vi "Tetra_TX-PROD_Payload.vi"(8 "error in":errorcluster, 10 "Input Constants":string[](array[string])=["18.75;1", "5;1", "COM4", "1", "1", "25", "0;0", "0;0", "1;20", "0", "0", "0", "", "10", "Z:\\State Files\\TEST2.csa", "", "3000", "4", "-10", "0.1", "", "", "C:\\RageATE\\Automated Tests\\Tetra WAM\\DVT\\Cal Files\\OUTPUT_CAL_080321-1118.csv"], 11 "Parameters":string[](array[string])=["skip", "18.75", "1", "5", "-1", "0", "5", "32.900000"]) -> (0 "error out":errorcluster, 2 "Payload Results":string[](array[string])=["-1.000", "-1.000", "32900.031", "-94.423", "-86.423", "-1.000", "16.450", "-1.000", "-1.000", "-1.000", "-1.000", "-1.000", "3.000", "-1.000", "-1.000", "15.000", "8.000", "8.000", "8.000", "-1.000", "-1.000", "-1.000", "-1.000", "-1.000", "-1.000", "-1.000", "-1.000", "-1.000", "-1.000", "-1.000", "-1.000", "-1.000", "-1.000", "-1.000", "-1.000", "-1.000", "-1.000", "-1.000", "-1.000", "-1.000", "-1.000", "-1.000", "-1.000", "-1.000", "0.504", "130.000", "-8.000", "32900.000", "-1.000", "-1.000", "P0027", "", "-1"])   [LabVIEW 2018]
uses:
  C:/RageATE-Tetra/Instruments/Ess Temp Plate/LabView Driver/Public/Watbus.dll
  Instruments/Ess Temp Plate/LabView Driver/Public/Watbus.dll
  8a334051-eedf-4406-ba3b-4766be56bf9e.vi
  458b4a15-084f-46bd-ad65-8d84519d0715.vi
  e7e3a4d5-9ed6-4285-8f90-f7af1205463a.vi
  778a857b-ea1c-4c41-85f0-8bde546241f8.vi
  765396e5-d7fa-4d1d-a6be-20604e030d46.vi
  35825170-2933-49a7-a6a3-6a45a8b9c174.vi
  498168d9-979f-4171-bbb2-b986919cd012.vi
  fd570da2-80e1-4258-b5ac-03cfe2f2c2d7.vi
  51f53847-2d88-46b1-9baf-ea88b261c08d.vi
  Infrastructure/Test Parameter Globals_1.0.0.vi
  Initialize References/Sequence Globals.vi
  Initialize References/Station References Global.vi
  Infrastructure/Test Result File Name Global.vi
  Tetra_Globals.vi
  <vilib>/Utility/file.llb/Write Delimited Spreadsheet (DBL).vi
  <vilib>/Utility/file.llb/Read Delimited Spreadsheet (DBL).vi
  Instruments/Agilent N5232A PNA-L/Labview Driver/Keysight PNA Series/Keysight PNA Series.lvlib
  Instruments/PNA/lib functions/Agilent ENA Series.lvlib
panel:
  out "result path":string
  out "adar_id":i32
  out "ser_rd":string
  out "AntiGlitch?(t)":bool
  in  "GetS11FromFile?(t)":bool=TRUE
  out "AVG_HARM":i32=4
  out "hx_fsl_corr":dbl=-1.0
  out "h2_fsl_corr":dbl=-1.0
  out "bypass ESA Freq Set(t)":bool
  out "TX-PASS?(T)":bool
  in  "Load_Prod_Limits(T)":bool=TRUE
  out "tx_flat_lim":dbl
  out "Tx_Flat":dbl
  out "resulting string":string
  out "TxFiltRead":bool
  out "x > 0?":bool
  in  "ess_error":errorcluster
  out "Freq Display":dbl=32.9 caption="Freq :  20"
  in  "Tab Control":T1(tab)
  out "MEAS_DCMON":bool
  out "CHIP_TEMP(t)":bool
  out "COMPORT":string="COM4"
  out "MODE":bool=TRUE
  out "Dist":dbl
  out "FILT_FCUT":dbl=25.0
  out "PLATE_TEMP(t)":bool
  out "MEAS_PS":bool
  out "MEAS_H2":bool=TRUE
  out "MEAS_Hx":bool=TRUE
  out "Hx_FREQ":dbl
  out "Hx_MULT":dbl
  out "H2_FREQ":dbl=40.0
  out "GANTRY(t)":bool=TRUE
  out "GET_DETECT":bool
  out "cmd;":string
  out "SOAK(m)":dbl
  out "Apply_FSL(t)":bool=TRUE
  out "MEAS_S11":bool
  out "S11_PORT":dbl
  out "comport":refnum<visa-resource-name>="COM4"
  out "AVG":i32=4
  out "ILabVIEW":refnum<k24>
  out "TEMP":dbl=25.0
  out "TX_PORT":i32=1
  out "V_SUPPLY":dbl=18.75
  out "EXT_ATT":dbl=5.0
  out "ADAR ATT":dbl
  out "TX_FILTER":i32=3
  out "REF_POW":dbl=5.0
  out "RF_FREQ":dbl=32.9
  out "TEMP(t)":bool
  out "V_SUPPLY(t)":bool
  out "TX_PORT(t)":bool
  out "REF_PWR(t)":bool
  out "TX_FILT(t)":bool
  out "ADAR_ATT(t)":bool
  out "EXT_ATT(t)":bool
  out "RF_FREQ(t)":bool=TRUE
  out "f_ref":dbl=16.45
  out "hx(t)":bool
  out "h2(t)":bool
  out "use-adar(t)":bool
  out "use-psa(t)":bool
  out "ps_meas(i)(w)":dbl[](array[numeric])=[-1.0, -1.0]
  out "rdv":dbl[](array[numeric])=[-1.0, -1.0, -1.0, -1.0, -1.0, -1.0, -1.0, -1.0, -1.0, -1.0]
  out "rdiv(i)":dbl[](array[numeric])=[-1.0, -1.0, -1.0, -1.0, -1.0, -1.0]
  out "rdiv(v)":dbl[](array[numeric])=[-1.0, -1.0, -1.0, -1.0, -1.0, -1.0]
  out "exa_mkr":dbl[](array[numeric])=[32900.0309, -94.423]
  out "h2_mkr":dbl[](array[numeric])=[-1.0, -1.0]
  out "Ampl_corr":dbl=-86.423
  out "s11":dbl=-1.0
  out "fsl_ampl_corr":dbl
  out "out_cal_ampl":dbl=-8.0
  out "out_cal freq":dbl=32900.0
  out "h2_dbc":dbl=-1.0
  out "hx_dbc":dbl
  out "hx_mkr":dbl[](array[numeric])
  out "fsl_corr_dB":dbl
  out "fsl(dB)":dbl
  out "hiband-flat":dbl
  out "lowband-flat":dbl
  out "h2_lim":dbl
  out "lowband-flat 2":dbl
  out "out_cal":dbl[][](array[numeric])=[[0.0, 0.0], [20000.0, -6.076], [20100.0, -6.075], [20200.0, -6.219], [20300.0, -6.234], [20400.0, -6.315], [20500.0, -6.131], [20600.0, -6.004], [20700.0, -6.283], [20800.0, -6.485], [20900.0, -6.42], [21000.0, -6.941], [21100.0, -6.789], [21200.0, -6.508], [21300.0, -6.41], [21400.0, -6.872], [21500.0, -6.938], [21600.0, -7.017], [21700.0, -7.269], [21800.0, -6.683], [21900.0, -6.297], [22000.0, -6.38], [22100.0, -6.432], [22200.0, -6.851], [22300.0, -6.503], [22400.0, -6.961], [22500.0, -6.827], [22600.0, -6.62], [22700.0, -6.74], [22800.0, -6.547], [22900.0, -6.559], [23000.0, -6.434], [23100.0, -6.642], [23200.0, -6.654], [23300.0, -6.563], [23400.0, -6.6], [23500.0, -6.836], [23600.0, -6.685], [23700.0, -6.139], [23800.0, -6.472], [23900.0, -6.849], [24000.0, -6.765], [24100.0, -6.802], [24200.0, -6.636], [24300.0, -6.397], [24400.0, -6.33], [24500.0, -6.799], [24600.0, -6.985], [24700.0, -7.181], [24800.0, -7.304], [24900.0, -7.242], [25000.0, -7.104], [25100.0, -7.249], [25200.0, -7.246], [25300.0, -7.161], [25400.0, -7.073], [25500.0, -7.471], [25600.0, -7.347], [25700.0, -7.254], [25800.0, -7.048], [25900.0, -7.016], [26000.0, -7.055], [26100.0, -7.436], [26200.0, -7.416], [26300.0, -7.406], [26400.0, -7.616], [26500.0, -7.56], [26600.0, -7.304], [26700.0, -7.165], [26800.0, -7.047], [26900.0, -7.196], [27000.0, -8.144], [27100.0, -7.775], [27200.0, -7.683], [27300.0, -8.261], [27400.0, -7.702], [27500.0, -7.067], [27600.0, -7.418], [27700.0, -7.363], [27800.0, -7.557], [27900.0, -8.241], [28000.0, -7.789], [28100.0, -7.932], [28200.0, -7.422], [28300.0, -7.539], [28400.0, -7.363], [28500.0, -7.293], [28600.0, -7.623], [28700.0, -7.8], [28800.0, -7.603], [28900.0, -7.302], [29000.0, -7.428], [29100.0, -7.212], [29200.0, -7.395], [29300.0, -7.337], [29400.0, -7.17], [29500.0, -7.328], [29600.0, -7.393], [29700.0, -7.363], [29800.0, -7.396], [29900.0, -7.295], [30000.0, -7.448], [30100.0, -7.434], [30200.0, -7.524], [30300.0, -7.411], [30400.0, -7.422], [30500.0, -7.643], [30600.0, -7.707], [30700.0, -7.612], [30800.0, -7.742], [30900.0, -7.916], [31000.0, -7.904], [31100.0, -8.064], [31200.0, -8.185], [31300.0, -8.079], [31400.0, -8.102], [31500.0, -8.357], [31600.0, -7.974], [31700.0, -8.361], [31800.0, -8.902], [31900.0, -8.745], [32000.0, -8.522], [32100.0, -8.392], [32200.0, -8.221], [32300.0, -7.885], [32400.0, -8.215], [32500.0, -8.486], [32600.0, -8.735], [32700.0, -8.287], [32800.0, -8.037], [32900.0, -8.0], [33000.0, -7.651], [33100.0, -7.755], [33200.0, -8.158], [33300.0, -8.086], [33400.0, -8.531], [33500.0, -8.093], [33600.0, -7.791], [33700.0, -7.841], [33800.0, -8.085], [33900.0, -7.787], [34000.0, -7.696], [34100.0, -8.068], [34200.0, -8.028], [34300.0, -7.958], [34400.0, -7.778], [34500.0, -8.182], [34600.0, -7.565], [34700.0, -7.759], [34800.0, -7.899], [34900.0, -7.536], [35000.0, -7.873], [35100.0, -8.126], [35200.0, -8.061], [35300.0, -7.731], [35400.0, -7.575], [35500.0, -7.802], [35600.0, -7.335], [35700.0, -7.39], [35800.0, -7.975], [35900.0, -7.981], [36000.0, -7.422], [36100.0, -7.632], [36200.0, -8.267], [36300.0, -7.907], [36400.0, -7.609], [36500.0, -7.858], [36600.0, -8.426], [36700.0, -8.44], [36800.0, -8.438], [36900.0, -8.536], [37000.0, -8.361], [37100.0, -8.731], [37200.0, -8.549], [37300.0, -8.609], [37400.0, -8.746], [37500.0, -9.42], [37600.0, -9.062], [37700.0, -8.792], [37800.0, -8.948], [37900.0, -8.893], [38000.0, -9.551], [38100.0, -9.086], [38200.0, -8.754], [38300.0, -8.61], [38400.0, -8.629], [38500.0, -8.895], [38600.0, -8.79], [38700.0, -8.437], [38800.0, -8.982], [38900.0, -8.564], [39000.0, -8.456], [39100.0, -8.944], [39200.0, -9.606], [39300.0, -9.246], [39400.0, -9.208], [39500.0, -9.78], [39600.0, -9.779], [39700.0, -9.292], [39800.0, -9.924], [39900.0, -9.871], [40000.0, -9.839]]
  out "h2_cal_ampl":dbl=-1.0
  out "h2_cal freq":dbl=-1.0
  out "h2_corr":dbl=-1.0
  out "h2_fsl_ampl_corr":dbl
  out "hx_cal_ampl":dbl=-1.0
  out "hx_cal freq":dbl=-1.0
  out "hx_fsl_ampl_corr":dbl
  out "hx_corr":dbl
  out "horn_Cal Freq Out":dbl
  out "horn_Ampl Out":dbl
  out "horn_cal":dbl[][](array[numeric])
  out "bpf":i32=1
  out "temp 0x":string="-1"
  out "detect":dbl=-1.0
  out "filt(num)":i32=3
  out "txatten-sel":i32=-1
  out "ext-atten(val)":dbl=-1.0
  out "adar-att(val)":dbl=-1.0
  out "iteration time(s)":dbl=91659.4314544 format="%_19f"
  out "relative seconds":dbl=91658.92763549999 format="%_19f"
  out "x-y":dbl=0.1592017999937525
  out "atten(code)ary (ro)":i32[](array[numeric])=[15, 8, 8, 8]
  out "plate_temp":sgl[](array[numeric])=[-1.0, -1.0] format="%.3g"
  out "temp_data":dbl[](array[numeric])
  out "readback":string
  out "dcw_lsl":dbl
  out "dcw_hsl":dbl
  out "pout_lsl":dbl
  out "pout_hsl":dbl
  out "s11_lsl":dbl
  out "s11_hsl":dbl
  out "FH_NOT(T)":bool
  out "no_fault":bool
  out "STOP(T)":bool
  out "pna-att":dbl=20.0
  out "do cmd?(f)":bool
  out "txp_#ofretries":i32
  # "Constants Locals Used in Payload"
  # "Index\tKey\tInput Constants\tUnits\n0\t1\tPS1-1 V;I\tVolt : Amp\n1\t1\tPS1-2 V:I\tVolt : Amp\n2\t1\tCOM PORT\tSTR\n3\t1\tMODE\tBool\n4\t1\tTXPORT;Antenna Dist\tant/inch\n5\t1\tTX Filt Cutoff\tGHz\n6\t1\tMeas Plate Temp; Meas Chip Temp\tBool;Bool\n7\t1\tMeas DC PS;Meas DCMON (Chip)\tBool;Bool\n8\t1\tMeas H2 \tBool;Freq(GHz)\n9\t1\tMeas H*x\tFreq(GHz);multiplier\n10\t1\tMeas S11;TXPORT\tBool;num\n11\t1\tRead Detector (1-4) \tBool\n12\t1\tcmd;…\tcmd;cmd\n13\t1\tTemp Soak Time\tmin\n14\t1\tPNA State File (local)\tPath\n15\t1\tENA State File\tPath\n16\t1\tENA RBW\tHz\n17\t1\tENA #of AVGs\tnum\n18\t1\tENA Ref Lvl\tdB\n19\t1\tENA Span\tMHz\n20\t1\tRFIN_CAL\tpath\n21\t1\tHORN_CAL\tpath\n22\t1\tOUTPUT_CAL\tpath\n23\t1\tFSL_APPLY\tbool\n24\t1\tDCW_LIMITS\tlsl;hsl\n25\t1\tPOUT_LIMITS\tlsl;hsl\n26\t1\tS11_LIMITS\tlsl;hsl"
  # "Input Parameters Locals"
  # "Update(t)"
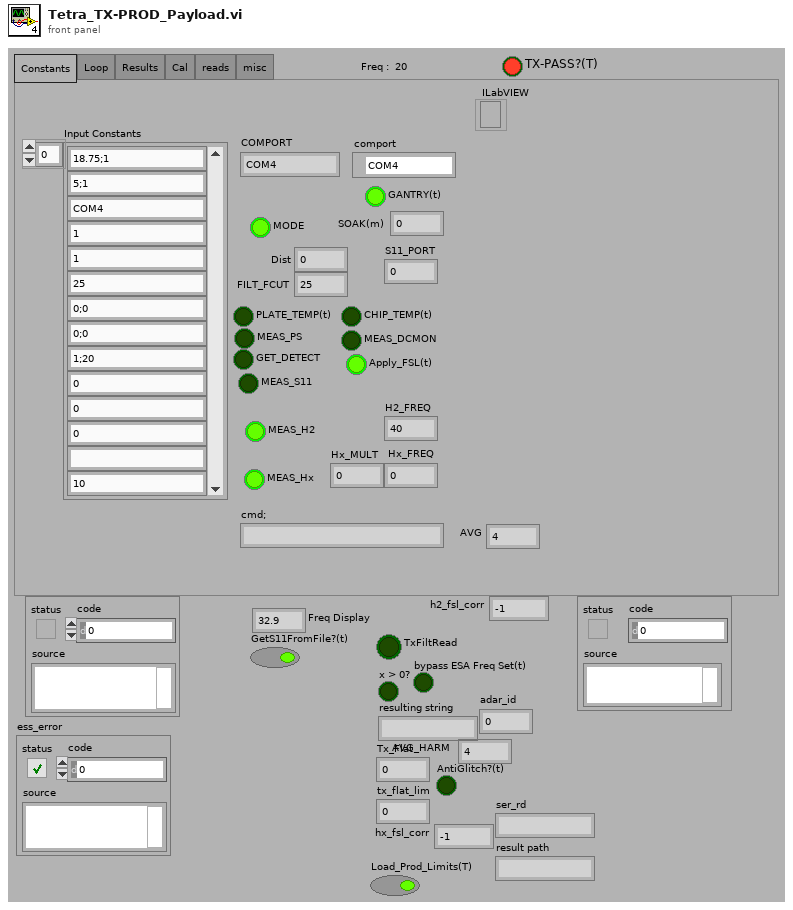
[diagram p1: front panel]
types:
  T1 = enum32{"Constants", "Loop", "Results", "Cal", "reads", "misc"}
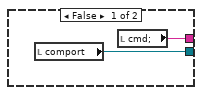
[diagram p3: hidden frame]
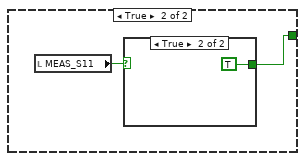
[diagram p4: hidden frame]
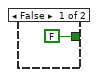
[diagram p5: hidden frame]
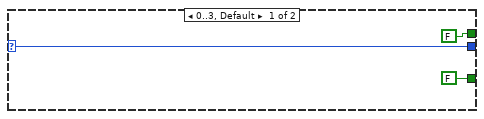
[diagram p6: hidden frame]
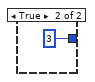
[diagram p7: hidden frame]
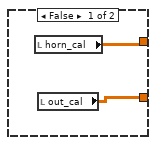
[diagram p8: hidden frame]
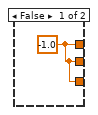
[diagram p9: hidden frame]
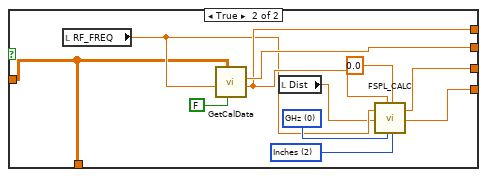
[diagram p10: hidden frame]
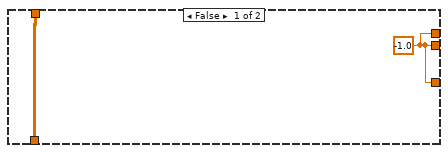
[diagram p11: hidden frame]
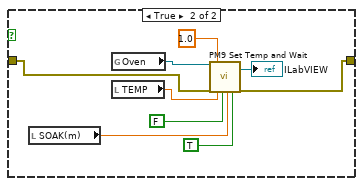
[diagram p12: hidden frame]
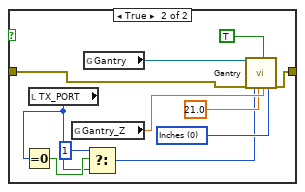
[diagram p13: hidden frame]
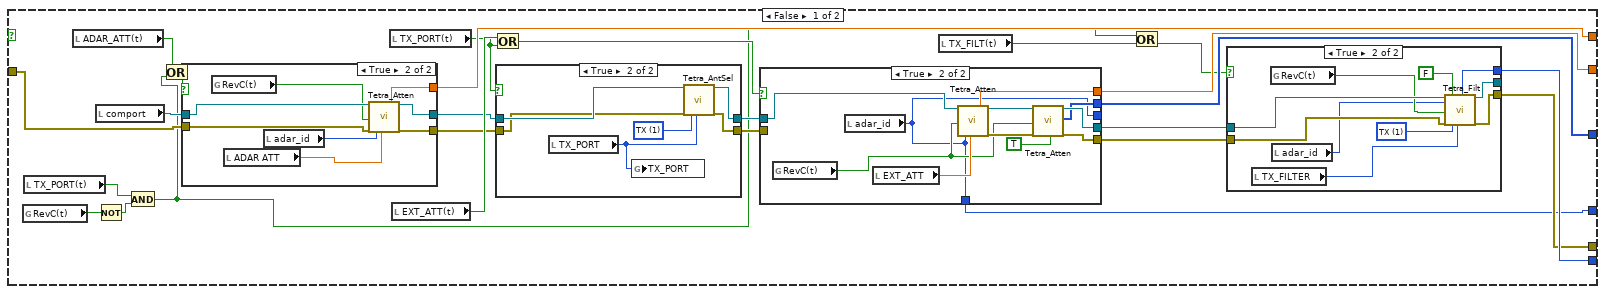
[diagram p15: hidden frame]
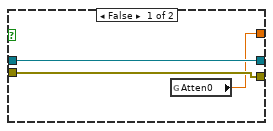
[diagram p17: hidden frame]
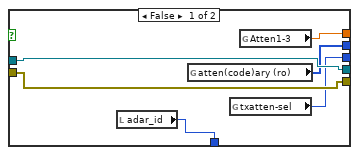
[diagram p18: hidden frame]
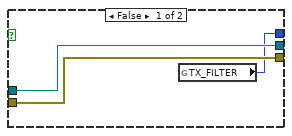
[diagram p19: hidden frame]
diagram:
  # "70\t1\tdc_hsl\tWatt\n71\t1\tdc_lsl\tWatt\n72\t1\tp_out_hsl\tdBm\n73\t1\tp_out_lsl\tdBm\n74\t1\ts11_hsl\tdb\n75\t1\ts11_lsl\tdb\n76\t1\th2_lim\tdbc\n77\t1\tdc|pout|s11|h2 (p/f)\t4b  bool \n78\t1\tpass/fail\tBool\n79\t1\tess_fault\tBool"
  n1 = flat-sequence {
    tunnel: ["error in"] -> w18
    tunnel: [w47] -> w20
    tunnel: [w46] -> w19
    tunnel: w18 -> [w44]
    tunnel: w20 -> [w1152]
    tunnel: w19 -> [w1132]
    tunnel: [w1152] -> w17
    tunnel: [w1132] -> w16
    tunnel: [w1145] -> w15
    tunnel: [w1144] -> w14
    tunnel: [w1143] -> w13
    tunnel: [w1151] -> w12
    tunnel: [w1150] -> w11
    tunnel: [w1149] -> w10
    tunnel: [w1148] -> w9
    tunnel: [w1147] -> w8
    tunnel: [w1146] -> w7
    tunnel: [w1142] -> w6
    tunnel: [w1141] -> w5
    tunnel: [w1130] -> w4
    tunnel: [w1129] -> w3
    tunnel: [w1128] -> w2
    tunnel: [w1127] -> w1
    tunnel: w17 -> [w1408]
    tunnel: w16 -> [w1395]
    tunnel: w15 -> [w1391]
    tunnel: w14 -> [w1406]
    tunnel: w13 -> [w1407]
    tunnel: w12 -> [w1405]
    tunnel: w11 -> [w1404]
    tunnel: w10 -> [w1403]
    tunnel: w9 -> [w1401]
    tunnel: w8 -> [w1400]
    tunnel: w7 -> [w1399]
    tunnel: w6 -> [w1402]
    tunnel: w5 -> [w1398]
    tunnel: w4 -> [w1393]
    tunnel: w3 -> [w1389]
    tunnel: w2 -> [w1386]
    tunnel: w1 -> [w1382]
    frame #0 {
      # "REV-C_TETRA_TX-PROD-DVT_LowRef"
      n2 = flat-sequence {
        frame #0 {
          w33 = TRUE ("Test Running (T)")
          n3 = global read "Station References Global.vi" "Gantry"() -> (w34:refnum<visa-resource-name>)
          n4 = call "WAM_ESS.vi"("VISA resource name"=w34, "error in (no error)"="ess_error", "Open Serial"=w33, "Test Running (T)"=w33, "Close Serial"=w33) -> ("FH_NOT(T)"=→"FH_NOT(T)":bool, "error out"=w31:errorcluster)  [unwired: 7 in, 2 out]
          n5 = local write "ess_error"(w31) -> ()
        }
      }
      n6 = global read "Test Result File Name Global.vi" "Test Results File Name"() -> (w22:path)
      n7 = First Call?() -> (First Call?: T/F=w23:bool)
      n8 = global read "Test Parameter Globals_1.0.0.vi" "Test Name"() -> (w28:string)
      n9 = And(x="Load_Prod_Limits(T)", y=w23) -> (x .and. y?=w25:bool)
      n10 = case shown="True" w25 {
        frame False {
        }
        frame True {
          n11 = global read "Sequence Globals.vi" "DevSupportPath"() -> (w38:path)
          n12 = global read "Sequence Globals.vi" "AppSupportPath 2"() -> (w40:path)
          n13 = global read "Sequence Globals.vi" "IsRuntime?"() -> (w41:bool)
          n14 = Build Path(base path=w38, name or relative path=path "3500007_TetraFinalTestAnalysis/testreport.ini" ("*.ini file")) -> (appended path=w36:path)
          n15 = Strip Path(path=w36) -> (name=w42:string)  [unwired: 1 out]
          n16 = Build Path(base path=w40, name or relative path=w42) -> (appended path=w39:path)
          n17 = Select(t=w39, s=w41, f=w36) -> (s? t:f=w43:path)
          n18 = call "ProdLimits.vi"("*.ini file"=w43) -> ()  [unwired: 9 in, 2 out]
        }
      }
      n19 = Path To String(path=w22) -> (string=→"result path":string)
      n20 = Equal?(x=w28, y="REV-C_TETRA_TX-PROD-DVT_LowRef") -> (x = y?=→"bypass ESA Freq Set(t)":bool)
      n21 = local write "TX-PASS?(T)"(FALSE ("TX-PASS?(T)")) -> ()
    }
    frame #1 {
      n22 = for {
        N: 2 -> [_]
        tunnel: [w58] -> w47
        tunnel: [w57] -> w46
        tunnel: w44 -> [w56]
        i -> [w53]
        stop <- w51 stop-if-true
        n23 = flat-sequence {
          tunnel: [w90] -> w89
          tunnel: ["Parameters"] -> w88
          tunnel: ["Input Constants"] -> w87
          tunnel: w56 -> [w90]
          tunnel: w89 -> [w95]
          tunnel: [w94] -> w86
          tunnel: w88 -> [w108]
          tunnel: w87 -> [w107]
          tunnel: [w106] -> w85
          tunnel: [w105] -> w84
          tunnel: [w104] -> w83
          tunnel: [w103] -> w82
          tunnel: [w102] -> w81
          tunnel: [w100] -> w80
          tunnel: [w101] -> w79
          tunnel: [w99] -> w78
          tunnel: [w98] -> w77
          tunnel: [w97] -> w76
          tunnel: w86 -> [w250]
          tunnel: [w250] -> w75
          tunnel: w85 -> [w249]
          tunnel: w84 -> [w246]
          tunnel: w83 -> [w234]
          tunnel: w82 -> [w229]
          tunnel: w81 -> [w243]
          tunnel: w80 -> [w242]
          tunnel: w79 -> [w240]
          tunnel: w78 -> [w237]
          tunnel: w77 -> [w235]
          tunnel: w76 -> [w227]
          tunnel: w75 -> [w303]
          tunnel: [w302] -> w74
          tunnel: [w383] -> w73
          tunnel: w74 -> [w382]
          tunnel: w73 -> [w399]
          tunnel: [w399] -> w72
          tunnel: w72 -> [w401]
          tunnel: [w401] -> w55
          tunnel: [w419] -> w71
          tunnel: w55 -> [w419]
          tunnel: w71 -> [w420]
          tunnel: [w421] -> w70
          tunnel: w70 -> [w433]
          tunnel: [w433] -> w69
          tunnel: [w432] -> w68
          tunnel: [w436] -> w67
          tunnel: w69 -> [w435]
          tunnel: w68 -> [w434]
          tunnel: [w434] -> w66
          tunnel: w67 -> [w604]
          tunnel: [w603] -> w65
          tunnel: w66 -> [w608]
          tunnel: [w617] -> w64
          tunnel: w65 -> [w616]
          tunnel: w64 -> [w641]
          tunnel: [w641] -> w63
          tunnel: w63 -> [w647]
          tunnel: [w642] -> w62
          tunnel: [w901] -> w61
          tunnel: w62 -> [w903]
          tunnel: w61 -> [w1004]
          tunnel: [w1004] -> w60
          tunnel: [w1006] -> w59
          tunnel: w60 -> [w1005]
          tunnel: w59 -> [w1037]
          tunnel: [w1037] -> w49
          tunnel: [w1036] -> w54
          tunnel: w49 -> [w1062]
          tunnel: [w1061] -> w48
          tunnel: [w1092] -> w58
          tunnel: w48 -> [w1079]
          tunnel: [w1080] -> w57
          tunnel: [w1081] -> w50
          frame #0 {
            n24 = call <vilib>:"High Resolution Relative Seconds.vi"() -> ("relative seconds"=→"relative seconds":dbl)
          }
          frame #1 {
            n25 = flat-sequence {
              tunnel: w107 -> [w212]
              tunnel: [w181] -> w97
              frame #0 {
                w140 = ";" ("regular expression")
                # "Get the Test Constants"
                n26 = Index Array(array=w212, index #1=2 ("index"), index #3=4 ("index"), index #8=10 ("index"), index #10=17 ("index"), index #11=20 ("index"), index #12=9 ("index"), index #13=13 ("index"), index #14=23 ("index")) -> (element #1=→"COMPORT":string, element #2=w187:string, element #3=w163:string, element #4=w202:string, element #5=w206:string, element #6=w205:string, element #7=w196:string, element #8=w185:string, element #9=w197:string, element #10=w141:string, element #12=w179:string, element #13=w168:string, element #14=w164:string, element #15=w155:string, element #16=w158:string, element #17=w150:string, element #18=w144:string, element #19=w143:string, element #20=→"ser_rd":string)  [unwired: 12 in, 1 out]
                n27 = call "StringToNumberControlWithBool.vi"("String In"=w187) -> ("NOT = 0"=→"MODE":bool)  [unwired: 7 in, 1 out]
                n28 = call "StringToNumberControlWithBool.vi"("String In"=w202) -> ("Number Out"=→"FILT_FCUT":dbl)  [unwired: 7 in, 1 out]
                n29 = call "StringToNumberControlWithBool.vi"("String In"=w197) -> ("NOT = 0"=→"GET_DETECT":bool)  [unwired: 7 in, 1 out]
                n30 = call "StringToNumberControlWithBool(x2).vi"("Seperator"=w140, "string"=w141) -> ("Num(2)"=→"AVG_HARM":dbl, "Num"=→"AVG":dbl)  [unwired: 3 in, 5 out]
                n31 = call "StringToNumberControlWithBool.vi"("String In"=w168) -> ("Number Out"=→"SOAK(m)":dbl)  [unwired: 7 in, 1 out]
                n32 = call "StringToNumberControlWithBool.vi"("String In"=w143) -> ("Number Out"=→"tx_flat_lim":dbl)  [unwired: 7 in, 1 out]
                n33 = call <vilib>:"Trim Whitespace.vi"("string"=w179) -> ("trimmed string"=w175:string)  [unwired: 1 in]
                n34 = Match Pattern(string=w163, regular expression=";") -> (before substring=w162:string, after substring=w160:string)  [unwired: 1 in, 2 out]
                n35 = Match Pattern(string=w206, regular expression=";") -> (before substring=w210:string, after substring=w209:string)  [unwired: 1 in, 2 out]
                n36 = Match Pattern(string=w205, regular expression=";") -> (before substring=w218:string, after substring=w217:string)  [unwired: 1 in, 2 out]
                n37 = Match Pattern(string=w196, regular expression=";") -> (before substring=w194:string, after substring=w192:string)  [unwired: 1 in, 2 out]
                n38 = Match Pattern(string=w185, regular expression=w140) -> (before substring=w184:string, after substring=w182:string)  [unwired: 1 in, 2 out]
                n39 = call "StringToNumberControlWithBool(x2).vi"("Seperator"=";" ("regular expression"), "string"=w155) -> ("Num(2)"=→"dcw_hsl":dbl, "Num"=→"dcw_lsl":dbl, "Seperator Out"=w151:string)  [unwired: 3 in, 4 out]
                n40 = Empty String/Path?(string/path=w182) -> (empty?=w181:bool)
                n41 = call "StringToNumberControlWithBool.vi"("String In"=w162) -> ("NOT = 0"=→"GANTRY(t)":bool)  [unwired: 7 in, 1 out]
                n42 = call "StringToNumberControlWithBool.vi"("String In"=w160) -> ("Number Out"=→"Dist":dbl)  [unwired: 7 in, 1 out]
                n43 = call "StringToNumberControlWithBool.vi"("String In"=w210) -> ("NOT = 0"=→"PLATE_TEMP(t)":bool)  [unwired: 7 in, 1 out]
                n44 = call "StringToNumberControlWithBool.vi"("String In"=w209) -> ("NOT = 0"=→"CHIP_TEMP(t)":bool)  [unwired: 7 in, 1 out]
                n45 = call "StringToNumberControlWithBool.vi"("String In"=w218) -> ("NOT = 0"=→"MEAS_PS":bool)  [unwired: 7 in, 1 out]
                n46 = call "StringToNumberControlWithBool.vi"("String In"=w217) -> ("NOT = 0"=→"MEAS_DCMON":bool)  [unwired: 7 in, 1 out]
                n47 = call "StringToNumberControlWithBool.vi"("String In"=w194) -> ("NOT = 0"=→"MEAS_H2":bool)  [unwired: 7 in, 1 out]
                n48 = call "StringToNumberControlWithBool.vi"("String In"=w192) -> ("Number Out"=→"H2_FREQ":dbl)  [unwired: 7 in, 1 out]
                n49 = call "StringToNumberControlWithBool.vi"("String In"=w184) -> ("NOT = 0"=→"MEAS_S11":bool)  [unwired: 7 in, 1 out]
                n50 = call "StringToNumberControlWithBool.vi"("String In"=w182) -> ("Number Out"=→"S11_PORT":dbl)  [unwired: 7 in, 1 out]
                n51 = call "StringToNumberControlWithBool(x2).vi"("Seperator"=w151, "string"=w158) -> ("Num(2)"=→"pout_hsl":dbl, "Num"=→"pout_lsl":dbl, "Seperator Out"=w149:string)  [unwired: 3 in, 4 out]
                n52 = Match Pattern(string=w175, regular expression=";") -> (before substring=w178:string, after substring=w177:string)  [unwired: 1 in, 2 out]
                n53 = call "StringToNumberControlWithBool.vi"("String In"=w178) -> ("Number Out"=→"Hx_FREQ":dbl, "NOT = 0"=w174:bool)  [unwired: 7 in]
                n54 = call "StringToNumberControlWithBool.vi"("String In"=w177) -> ("Number Out"=→"Hx_MULT":dbl, "NOT = 0"=w173:bool)  [unwired: 7 in]
                n55 = call "StringToNumberControlWithBool(x2).vi"("Seperator"=w149, "string"=w150) -> ("Num(2)"=→"s11_hsl":dbl, "Num"=→"s11_lsl":dbl, "Seperator Out"=w146:string)  [unwired: 3 in, 4 out]
                n56 = And(x=w174, y=w173) -> (x .and. y?=→"MEAS_Hx":bool)
                n57 = call "StringToNumberControlWithBool(x2).vi"("Seperator"=w146, "string"=w144) -> ("Num"=→"h2_lim":dbl)  [unwired: 3 in, 6 out]
                n58 = call "StringToNumberControlWithBool.vi"("String In"=w164) -> ("NOT = 0"=→"Apply_FSL(t)":bool)  [unwired: 7 in, 1 out]
              }
            }
            n59 = control-ref of="Freq Display"() -> (w96:refnum<vi>)
            n60 = flat-sequence {
              tunnel: w108 -> [w135]
              tunnel: [w113] -> w106
              tunnel: [w112] -> w105
              tunnel: [w134] -> w104
              tunnel: [w133] -> w103
              tunnel: [w132] -> w102
              tunnel: [w131] -> w101
              tunnel: [w130] -> w100
              tunnel: [w128] -> w99
              tunnel: [w109] -> w98
              tunnel: w96 -> [w123]
              tunnel: w95 -> [w120]
              tunnel: [w119] -> w94
              frame #0 {
                # "Get the Test Parameters"
                n61 = Index Array(array=w135) -> (element #1=w130:string, element #2=w137:string, element #3=w136:string, element #4=w127:string, element #5=w126:string, element #6=w125:string, element #7=w118:string, element #8=w110:string)  [unwired: 9 in, 1 out]
                n62 = call "TempControlWithBool.vi"("INPUT"=w130) -> ("out"=→"TEMP":dbl, "Valid(t)"=w128:bool)  [unwired: 6 in, 1 out]
                n63 = Fract/Exp String To Number(string=w137) -> (number=w132:dbl)  [unwired: 3 in, 1 out]
                "V_SUPPLY" <- w132
                n64 = Decimal String To Number(string=w136) -> (number=w133:i32)  [unwired: 2 in, 1 out]
                "TX_PORT" <- w133
                n65 = Fract/Exp String To Number(string=w127) -> (number=w131:dbl)  [unwired: 3 in, 1 out]
                "REF_POW" <- w131
                n66 = Decimal String To Number(string=w126) -> (number=w134:i32)  [unwired: 2 in, 1 out]
                "TX_FILTER" <- w134
                n67 = Fract/Exp String To Number(string=w125) -> (number=w112:dbl)  [unwired: 3 in, 1 out]
                "ADAR ATT" <- w112
                n68 = Fract/Exp String To Number(string=w118) -> (number=w113:dbl)  [unwired: 3 in, 1 out]
                "EXT_ATT" <- w113
                n69 = Fract/Exp String To Number(string=w110) -> (number=w109:dbl)  [unwired: 3 in, 1 out]
                "RF_FREQ" <- w109
                "Freq Display" <- w109
                n70 = Concatenate Strings("Freq :  " ("string"), w110) -> (w122:string)
                n71 = Divide(x=w109, y=2.0) -> (x/y=→"f_ref":dbl)
                n72 = Not Equal?(x=w112, y=-1.0) -> (x != y?=→"use-adar(t)":bool)
                n73 = Not Equal?(x=w113, y=-1.0) -> (x != y?=→"use-psa(t)":bool)
                n74 = property class="DigNum (strict)"(reference=w123, error in=w120, "Caption.Text"=w122) -> (error out=w119:errorcluster)  [unwired: 1 out]
              }
            }
          }
          frame #2 {
            # "Check if value changed\nif value changed (t) use to skip the routine"
            n75 = call "Is Value Changed.vim"("value"=w242) -> ("changed or first call?"=w239:bool)
            n76 = call "Is Value Changed.vim"("value"=w243) -> ("changed or first call?"=→"V_SUPPLY(t)":bool)
            n77 = call "Is Value Changed.vim"("value"=w229) -> ("changed or first call?"=→"TX_PORT(t)":bool)
            n78 = call "Is Value Changed.vim"("value"=w240) -> ("changed or first call?"=→"REF_PWR(t)":bool)
            n79 = call "Is Value Changed.vim"("value"=w246) -> ("changed or first call?"=→"ADAR_ATT(t)":bool)
            n80 = call "Is Value Changed.vim"("value"=w249) -> ("changed or first call?"=→"EXT_ATT(t)":bool)
            n81 = call "Is Value Changed.vim"("value"=w235) -> ("changed or first call?"=→"RF_FREQ(t)":bool)
            n82 = flat-sequence {
              frame #0 {
                # "Setup the H2 measurement"
                n83 = local read "RF_FREQ"() -> (w280:dbl)
                n84 = local read "H2_FREQ"() -> (w276:dbl)
                n85 = local read "MEAS_H2"() -> (w277:bool)
                n86 = Equal?(x=w276, y=w280) -> (x = y?=w279:bool)
                n87 = Multiply(x=w276, y=2.0) -> (x*y=w274:dbl)
                n88 = And(x=w279, y=w277) -> (x .and. y?=→"h2(t)":bool)
                n89 = local write "H2_FREQ"(w274) -> ()
              }
            }
            n90 = case shown="-1" w234 {
              selector: w234 -> [w283 _]
              tunnel: [w283 w286] -> w233
              tunnel: [FALSE ("changed or first call?") w285] -> w230
              tunnel: [FALSE ("TxFiltRead") TRUE ("TxFiltRead")] -> w222
              frame 0..3, Default {
              }
              frame -1 {
                n91 = local read "FILT_FCUT"() -> (w288:dbl)
                n92 = local read "RF_FREQ"() -> (w289:dbl)
                n93 = Greater Or Equal?(x=w289, y=w288) -> (x >= y?=w287:bool)
                n94 = case shown="False" w287 {
                  tunnel: [2 3] -> w286
                  frame False {
                  }
                  frame True {
                  }
                }
                n95 = call "Is Value Changed.vim"("value"=w286) -> ("changed or first call?"=w285:bool)
              }
            }
            "TxFiltRead" <- w222
            n96 = flat-sequence {
              frame #0 {
                # "Setup the H*X measurement"
                n97 = local read "RF_FREQ"() -> (w264:dbl)
                n98 = local read "Hx_MULT"() -> (w258:dbl)
                n99 = local read "Hx_FREQ"() -> (w260:dbl)
                n100 = local read "MEAS_Hx"() -> (w261:bool)
                n101 = Multiply(x=w260, y=w258) -> (x*y=w259:dbl)
                n102 = Equal?(x=w260, y=w264) -> (x = y?=w263:bool)
                n103 = And(x=w263, y=w261) -> (x .and. y?=→"hx(t)":bool)
                n104 = local write "Hx_FREQ"(w259) -> ()
              }
            }
            n105 = local read "MEAS_S11"() -> (w225:bool)
            n106 = First Call?() -> (First Call?: T/F=w223:bool)
            n107 = case shown="True" w223 {
              tunnel: [w252 w257] -> w220
              tunnel: [w251 w253] -> w224
              frame False {
                n108 = local read "comport"() -> (w251:refnum<visa-resource-name>)
                n109 = local read "cmd;"() -> (w252:string)
              }
              frame True {
                n110 = local read "COMPORT"() -> (w254:string)
                n111 = global read "Tetra_Globals.vi" "comport"() -> (w255:refnum<visa-resource-name>)
                n112 = Empty String/Path?(string/path=w254) -> (empty?=w256:bool)
                n113 = Select(t=w255, s=w256, f=w254) -> (s? t:f=w253:refnum<visa-resource-name>)
                n114 = global read "Tetra_Globals.vi" "cmd;"() -> (w257:string)
              }
            }
            "cmd;" <- w220
            "comport" <- w224
            n115 = And(x=w239, y=w237) -> (x .and. y?=→"TEMP(t)":bool)
            n116 = And(x=w227, y=w225) -> (x .and. y?=w226:bool)
            n117 = case shown="False" w226 {
              tunnel: w229 -> [w269 _]
              tunnel: [w265 w271] -> w228
              frame False {
                n118 = local read "S11_PORT"() -> (w268:dbl)
                n119 = local read "MEAS_S11"() -> (w266:bool)
                n120 = Equal?(x=w268, y=w269) -> (x = y?=w267:bool)
                n121 = And(x=w266, y=w267) -> (x .and. y?=w265:bool)
              }
              frame True {
                n122 = local read "MEAS_S11"() -> (w270:bool)
                n123 = case shown="True" w270 {
                  tunnel: [FALSE TRUE] -> w271
                  frame False {
                  }
                  frame True {
                  }
                }
              }
            }
            n124 = call "Is Value Changed.vim"("value"=w234) -> ("changed or first call?"=w231:bool)
            n125 = Empty String/Path?(string/path=w220) -> (empty?=→"do cmd?(f)":bool)
            n126 = Or(x=w230, y=w231) -> (x .or. y?=→"TX_FILT(t)":bool)
            n127 = local write "TX_FILTER"(w233) -> ()
            n128 = local write "MEAS_S11"(w228) -> ()
          }
          frame #3 {
            n129 = flat-sequence "CALIBRATION TABLES" {
              tunnel: [w325] -> w302
              tunnel: w303 -> [w326]
              tunnel: [w304] -> w301
              tunnel: [w320] -> w300
              tunnel: [w319] -> w299
              tunnel: [w318] -> w298
              tunnel: [w317] -> w297
              tunnel: [w316] -> w296
              tunnel: [w315] -> w295
              tunnel: [w314] -> w294
              tunnel: [w313] -> w293
              tunnel: [w312] -> w292
              frame #0 {
                n130 = First Call?() -> (First Call?: T/F=w305:bool)
                n131 = case shown="True" w305 {
                  tunnel: [w331 w334] -> w322
                  tunnel: [w332 w333] -> w311
                  frame False {
                    n132 = local read "horn_cal"() -> (w332:dbl[][])
                    n133 = local read "out_cal"() -> (w331:dbl[][])
                  }
                  frame True {
                    n134 = global read "Tetra_Globals.vi" "HORN_CAL"() -> (w333:dbl[][])
                    n135 = global read "Tetra_Globals.vi" "OUT_CAL"() -> (w334:dbl[][])
                  }
                }
                "out_cal" <- w322
                "horn_cal" <- w311
                n136 = local read "RF_FREQ"() -> (w330:dbl)
                n137 = Multiply(x=w330, y=1000.0) -> (x*y=w329:dbl)
                n138 = call "GetCalData.vi"("Open new file T"=FALSE, "Ary In"=w322, "error in (no error)"=w326, "RF Freq (MHz)"=w329) -> ("error out"=w325:errorcluster, "Ampl Out"=→"out_cal_ampl":dbl, "Cal Freq Out"=→"out_cal freq":dbl, "array out"=w321:dbl[][])  [unwired: 2 in, 2 out]
                n139 = local read "Apply_FSL(t)"() -> (w308:bool)
                n140 = local read "MEAS_Hx"() -> (w306:bool)
                n141 = local read "MEAS_H2"() -> (w307:bool)
                n142 = case shown="False" w308 {
                  tunnel: [-1.0 ("Cal Freq Out") w363] -> w312
                  tunnel: [w352 w362] -> w313
                  tunnel: w311 -> [w351 w354]
                  tunnel: [w352 w358] -> w314
                  tunnel: [w352 w356] -> w315
                  tunnel: [w351 w354] -> w309
                  frame False {
                    w352 = 0.0 ("Ampl Out")
                  }
                  frame True {
                    w359 = u16 2 items=["Meter", "Feet", "Inches"] ("d(units)")
                    w361 = u16 0 items=["GHz", "MHz"] ("f(units)")
                    n143 = local read "RF_FREQ"() -> (w357:dbl)
                    n144 = call "GetCalData.vi"("Open new file T"=FALSE, "Ary In"=w354, "RF Freq (MHz)"=w357) -> ("Ampl Out"=w362:dbl, "Cal Freq Out"=w363:dbl)  [unwired: 3 in, 4 out]
                    n145 = local read "Dist"() -> (w355:dbl)
                    n146 = call "FSPL_CALC.vi"("f"=w357, "d"=w355, "Ant1 Gain (dB)"=w362, "f(units)"=w361, "Ant2 Gain dB"=0.0 ("Ant1 Gain (dB)"), "d(units)"=w359) -> ("Corr(dB)"=w358:dbl, "fsl(dB)"=w356:dbl)  [unwired: 11 in, 1 out]
                  }
                }
                n147 = case shown="True" w307 {
                  tunnel: [w366 w381] -> w316
                  tunnel: [w366 w380] -> w317
                  tunnel: w321 -> [_ w378]
                  tunnel: [w366 w370] -> w320
                  tunnel: w309 -> [w365 w367]
                  tunnel: [w365 w367] -> w310
                  frame False {
                    w366 = -1.0 ("Ampl Out")
                  }
                  frame True {
                    w373 = u16 2 items=["Meter", "Feet", "Inches"] ("d(units)")
                    w374 = u16 0 items=["GHz", "MHz"] ("f(units)")
                    n148 = local read "H2_FREQ"() -> (w371:dbl)
                    n149 = call "GetCalData.vi"("Open new file T"=FALSE, "Ary In"=w367, "RF Freq (MHz)"=w371) -> ("Ampl Out"=w369:dbl)  [unwired: 3 in, 5 out]
                    n150 = local read "Dist"() -> (w375:dbl)
                    n151 = Multiply(x=1000.0 ("y"), y=w371) -> (x*y=w379:dbl)
                    n152 = call "GetCalData.vi"("Open new file T"=FALSE, "Ary In"=w378, "RF Freq (MHz)"=w379) -> ("Ampl Out"=w380:dbl, "Cal Freq Out"=w381:dbl)  [unwired: 3 in, 4 out]
                    n153 = call "FSPL_CALC.vi"("f"=w371, "d"=w375, "Ant1 Gain (dB)"=w369, "f(units)"=w374, "Ant2 Gain dB"=0.0, "d(units)"=w373) -> ("Corr(dB)"=w370:dbl)  [unwired: 11 in, 2 out]
                  }
                }
                n154 = case shown="True" w306 {
                  tunnel: [w335 w350] -> w318
                  tunnel: [w335 w349] -> w319
                  tunnel: w321 -> [_ w347]
                  tunnel: [w335 w339] -> w304
                  tunnel: w310 -> [_ w336]
                  frame False {
                    w335 = -1.0 ("Ampl Out")
                  }
                  frame True {
                    w342 = u16 2 items=["Meter", "Feet", "Inches"] ("d(units)")
                    w343 = u16 0 items=["GHz", "MHz"] ("f(units)")
                    n155 = local read "Hx_FREQ"() -> (w340:dbl)
                    n156 = call "GetCalData.vi"("Open new file T"=FALSE, "Ary In"=w336, "RF Freq (MHz)"=w340) -> ("Ampl Out"=w338:dbl)  [unwired: 3 in, 5 out]
                    n157 = local read "Dist"() -> (w344:dbl)
                    n158 = Multiply(x=1000.0 ("y"), y=w340) -> (x*y=w348:dbl)
                    n159 = call "GetCalData.vi"("Open new file T"=FALSE, "Ary In"=w347, "RF Freq (MHz)"=w348) -> ("Ampl Out"=w349:dbl, "Cal Freq Out"=w350:dbl)  [unwired: 3 in, 4 out]
                    n160 = call "FSPL_CALC.vi"("f"=w340, "d"=w344, "Ant1 Gain (dB)"=w338, "f(units)"=w343, "Ant2 Gain dB"=0.0, "d(units)"=w342) -> ("Corr(dB)"=w339:dbl)  [unwired: 11 in, 2 out]
                  }
                }
              }
            }
            "h2_cal freq" <- w296
            "h2_cal_ampl" <- w297
            "hx_cal freq" <- w298
            "hx_cal_ampl" <- w299
            "h2_fsl_corr" <- w300
            "hx_fsl_corr" <- w301
            "horn_Cal Freq Out" <- w292
            "horn_Ampl Out" <- w293
            "fsl_corr_dB" <- w294
            "fsl(dB)" <- w295
          }
          frame #4 {
            n161 = flat-sequence {
              tunnel: [w387] -> w383
              tunnel: w382 -> [w386]
              frame #0 {
                # "3-23-22\nneed to add bypass if ess is tripped so it wont set the temperature and soak"
                # "Set The Temperature"
                n162 = global read "Station References Global.vi" "Oven Present?"() -> (w384:bool)
                n163 = local read "TEMP(t)"() -> (w388:bool)
                n164 = And(x=w388, y=w384) -> (x .and. y?=w385:bool)
                n165 = case shown="False" w385 {
                  tunnel: [w389 w398] -> w387
                  tunnel: w386 -> [w389 w393]
                  frame False {
                  }
                  frame True {
                    n166 = local read "SOAK(m)"() -> (w390:dbl)
                    n167 = global read "Station References Global.vi" "Oven"() -> (w392:refnum<visa-resource-name>)
                    n168 = local read "TEMP"() -> (w397:dbl)
                    n169 = call "PM9 Set Temp and Wait.vi"("VISA"=w392, "Error In"=w393, "Accuracy +/-"=1.0, "Set Point"=w397, "RO(t)"=FALSE, "Min (-1 for cont.)"=w390, "close session(t)"=TRUE) -> ("session out"=→"ILabVIEW":refnum<k24>, "error out"=w398:errorcluster)  [unwired: 9 in, 2 out]
                  }
                }
              }
            }
          }
          frame #5 {
          }
          frame #6 {
            n170 = flat-sequence {
              tunnel: [w406] -> w400
              frame #0 {
                (unwired) FALSE
                # "Move The Gantry"
                n171 = local read "TX_PORT(t)"() -> (w405:bool)
                n172 = local read "GANTRY(t)"() -> (w404:bool)
                n173 = local read "ess_error"() -> (w402:errorcluster)
                n174 = And(x=w405, y=w404) -> (x .and. y?=w403:bool)
                n175 = case shown="False" w403 {
                  tunnel: w402 -> [w407 w418]
                  tunnel: [w407 w417] -> w406
                  frame False {
                  }
                  frame True {
                    w412 = u16 0 items=["Inches", "cm"] ("Zunits")
                    n176 = local read "TX_PORT"() -> (w409:i32)
                    n177 = Equal To 0?(x=w409) -> (x = 0?=w410:bool)
                    n178 = global read "Tetra_Globals.vi" "Gantry_Z"() -> (w414:dbl)
                    n179 = global read "Station References Global.vi" "Gantry"() -> (w415:refnum<visa-resource-name>)
                    n180 = Select(t=1, s=w410, f=w409) -> (s? t:f=w408:i32)
                    n181 = call "Gantry.vi"("COMPORT"=w415, "error in (no error)"=w418, "Antenna Select"=w408, "z ref"=21.0, "Write(reads antenna co-ords when off)"=TRUE, "z"=w414, "Zunits"=w412) -> ("error out"=w417:errorcluster)  [unwired: 12 in]
                  }
                }
              }
            }
            n182 = local write "ess_error"(w400) -> ()
          }
          frame #7 {
          }
          frame #8 {
            n183 = flat-sequence {
              tunnel: [w424] -> w421
              tunnel: w420 -> [w423]
              frame #0 {
                # "Program the Power Supply"
                n184 = local read "V_SUPPLY(t)"() -> (w422:bool)
                n185 = case shown="True" w422 {
                  tunnel: [w425 w427] -> w424
                  tunnel: w423 -> [w425 w426]
                  frame False {
                  }
                  frame True {
                    w430 = "PS1"  # SEL_PS
                    n186 = local read "V_SUPPLY"() -> (w429:dbl)
                    n187 = global read "Station References Global.vi" "PS1"() -> (w431:refnum<visa-resource-name>)
                    n188 = call "INST_PS_SET_VOLTAGE_LEVEL_4.0.0.vi"("Instrument Select (Output 1)"="1", "SEL_PS"=w430, "error in (no error)"=w426, "Voltage (0.0)"=w429, "VISA session"=w431) -> ("error out"=w427:errorcluster)  [unwired: 5 in, 1 out]
                  }
                }
              }
            }
          }
          frame #9 {
            n189 = call <vilib>:"High Resolution Relative Seconds.vi"() -> ("relative seconds"=w432:dbl)
          }
          frame #10 {
            n190 = flat-sequence {
              tunnel: [w447] -> w436
              tunnel: w435 -> [w438]
              frame #0 {
                # "Program the Settings"
                n191 = local read "TX_PORT"() -> (w440:i32)
                n192 = call "Port To Atten Map.vi"("Port"=w440, "error in"=w438) -> ("error out"=w439:errorcluster, "txatten-sel"=→"adar_id":i32)  [unwired: 8 in]
                n193 = local read "MODE"() -> (w446:bool)
                n194 = case shown="True" w446 {
                  tunnel: [w462 w546] -> w447
                  tunnel: w439 -> [w451 w532]
                  tunnel: [w470 w525] -> w443
                  tunnel: [w469 w524] -> w444
                  tunnel: [w463 i32[] [-1, -1, -1, -1] ("atten(code)ary (ro)")] -> w445
                  tunnel: [w464 -1 ("txatten-sel")] -> w442
                  tunnel: [w448 w522] -> w437
                  frame False {
                    n195 = global read "Tetra_Globals.vi" "RevC(t)"() -> (w454:bool)
                    n196 = local read "TX_PORT(t)"() -> (w455:bool)
                    n197 = local read "ADAR_ATT(t)"() -> (w468:bool)
                    n198 = local read "comport"() -> (w465:refnum<visa-resource-name>)
                    n199 = Not(x=w454) -> (.not. x?=w452:bool)
                    n200 = And(x=w455, y=w452) -> (x .and. y?=w449:bool)
                    n201 = Or(x=w468, y=w449) -> (x .or. y?=w453:bool)
                    n202 = case shown="True" w453 {
                      tunnel: w465 -> [w482 w491]
                      tunnel: [w483 w490] -> w459
                      tunnel: [w481 w487] -> w470
                      tunnel: w451 -> [w483 w485]
                      tunnel: [w482 w488] -> w458
                      frame False {
                        n203 = global read "Tetra_Globals.vi" "Atten0"() -> (w481:dbl)
                      }
                      frame True {
                        n204 = global read "Tetra_Globals.vi" "RevC(t)"() -> (w486:bool)
                        n205 = local read "ADAR ATT"() -> (w489:dbl)
                        n206 = local read "adar_id"() -> (w484:i32)
                        n207 = call "Tetra_Atten.vi"("COMPORT"=w491, "RevC(T)"=w486, "error in (no error)"=w485, "TxAtten(num)"=w484, "Atten(dB)"=w489) -> ("atten(value)"=w487:dbl, "comport"=w488:refnum<visa-resource-name>, "error out"=w490:errorcluster)  [unwired: 10 in, 2 out]
                      }
                    }
                    n208 = local read "TX_PORT(t)"() -> (w456:bool)
                    n209 = local read "EXT_ATT(t)"() -> (w467:bool)
                    n210 = Or(x=w467, y=w456) -> (x .or. y?=w457:bool)
                    n211 = case shown="True" w456 {
                      tunnel: w458 -> [w473 w480]
                      tunnel: w459 -> [w474 w479]
                      tunnel: [w474 w477] -> w461
                      tunnel: [w473 w476] -> w460
                      frame False {
                      }
                      frame True {
                        w478 = 1 items=["RX", "TX"] ("TX/RX")
                        n212 = local read "TX_PORT"() -> (w475:i32)
                        n213 = global write "Tetra_Globals.vi" "TX_PORT"(w475) -> ()
                        n214 = call "Tetra_AntSel.vi"("COMPORT"=w480, "error in (no error)"=w479, "RX/TX"=w478, "ANT(num)"=w475) -> ("comport"=w476:refnum<visa-resource-name>, "error out"=w477:errorcluster)  [unwired: 13 in, 1 out]
                      }
                    }
                    n215 = case shown="True" w457 {
                      tunnel: [w496 w501] -> w472
                      tunnel: [w497 w506] -> w471
                      tunnel: w461 -> [w496 _]
                      tunnel: [w494 w498] -> _
                      tunnel: [w495 w500] -> w469
                      tunnel: w460 -> [w497 w507]
                      tunnel: [w493 w504] -> w463
                      tunnel: [w492 w498] -> w448
                      frame False {
                        n216 = local read "adar_id"() -> (w492:i32)
                        n217 = global read "Tetra_Globals.vi" "atten(code)ary (ro)"() -> (w493:i32[])
                        n218 = global read "Tetra_Globals.vi" "txatten-sel"() -> (w494:i32)
                        n219 = global read "Tetra_Globals.vi" "Atten1-3"() -> (w495:dbl)
                      }
                      frame True {
                        n220 = global read "Tetra_Globals.vi" "RevC(t)"() -> (w499:bool)
                        n221 = local read "adar_id"() -> (w498:i32)
                        n222 = local read "EXT_ATT"() -> (w508:dbl)
                        n223 = call "Tetra_Atten.vi"("COMPORT"=w507, "RevC(T)"=w499, "TxAtten(num)"=w498, "Atten(dB)"=w508) -> ("atten(value)"=w500:dbl, "comport"=w505:refnum<visa-resource-name>, "error out"=w502:errorcluster)  [unwired: 11 in, 2 out]
                        n224 = call "Tetra_Atten.vi"("COMPORT"=w505, "RevC(T)"=w499, "error in (no error)"=w502, "RO(t)"=TRUE) -> ("comport"=w506:refnum<visa-resource-name>, "atten(code)ary (ro)"=w504:i32[], "error out"=w501:errorcluster)  [unwired: 11 in, 2 out]
                      }
                    }
                    n225 = local read "TX_FILT(t)"() -> (w466:bool)
                    n226 = Or(x=w449, y=w466) -> (x .or. y?=w450:bool)
                    n227 = case shown="True" w450 {
                      tunnel: w472 -> [w511 w513]
                      tunnel: w471 -> [w510 w521]
                      tunnel: [w510 w520] -> _
                      tunnel: [w511 w518] -> w462
                      tunnel: [w509 w516] -> w464
                      frame False {
                        n228 = global read "Tetra_Globals.vi" "TX_FILTER"() -> (w509:i32)
                      }
                      frame True {
                        w519 = 1 items=["RX", "TX"] ("RX/TX")
                        n229 = local read "TX_FILTER"() -> (w517:i32)
                        n230 = global read "Tetra_Globals.vi" "RevC(t)"() -> (w514:bool)
                        n231 = local read "adar_id"() -> (w512:i32)
                        n232 = call "Tetra_Filt.vi"("COMPORT"=w521, "ADAR-ID"=w512, "Rev-C(T)"=w514, "error in (no error)"=w513, "RO(t)"=FALSE, "RX/TX"=w519, "Filt(sel)"=w517) -> ("filt(num)"=w516:i32, "comport"=w520:refnum<visa-resource-name>, "error out"=w518:errorcluster)  [unwired: 10 in]
                      }
                    }
                  }
                  frame True {
                    # "Program the Settings"
                    n233 = local read "comport"() -> (w531:refnum<visa-resource-name>)
                    n234 = local read "RF_FREQ(t)"() -> (w528:bool)
                    n235 = local read "TX_PORT(t)"() -> (w554:bool)
                    n236 = local read "ADAR_ATT(t)"() -> (w552:bool)
                    n237 = local read "use-adar(t)"() -> (w544:bool)
                    n238 = case shown="True" w554 {
                      tunnel: w531 -> [w593 w602]
                      tunnel: w532 -> [w594 w601]
                      tunnel: [w594 w599] -> w529
                      tunnel: [w593 w597] -> w530
                      frame False {
                      }
                      frame True {
                        w595 = FALSE ("Close Ser(t)")
                        w600 = 1 items=["RX", "TX"] ("TX/RX")
                        n239 = global read "Tetra_Globals.vi" "RevC(t)"() -> (w596:bool)
                        n240 = local read "TX_PORT"() -> (w598:i32)
                        n241 = global write "Tetra_Globals.vi" "TX_PORT"(w598) -> ()
                        n242 = call "Tetra_AntSel.vi"("COMPORT"=w602, "REVC(T)"=w596, "error in (no error)"=w601, "RX/TX"=w600, "ANT(num)"=w598, "Open Ser(t)"=w595, "Close Ser(t)"=w595) -> ("comport"=w597:refnum<visa-resource-name>, "error out"=w599:errorcluster)  [unwired: 10 in, 1 out]
                      }
                    }
                    n243 = And(x=w552, y=w544) -> (x .and. y?=w551:bool)
                    n244 = And(x=w528, y=w544) -> (x .and. y?=w543:bool)
                    n245 = Or(x=w551, y=w543) -> (x .or. y?=w545:bool)
                    n246 = global read "Tetra_Globals.vi" "RevC(t)"() -> (w535:bool)
                    n247 = local read "TX_PORT(t)"() -> (w537:bool)
                    n248 = Not(x=w535) -> (.not. x?=w534:bool)
                    n249 = And(x=w537, y=w534) -> (x .and. y?=w533:bool)
                    n250 = Or(x=w545, y=w533) -> (x .or. y?=w538:bool)
                    n251 = case shown="True" w528 {
                      tunnel: w530 -> [w555 w559]
                      tunnel: [w556 w558] -> w526
                      tunnel: w529 -> [w556 w560]
                      tunnel: [w555 w557] -> w527
                      frame False {
                      }
                      frame True {
                        n252 = disable-structure shown="Enabled" {
                          disable-tunnel: w560 -> [w567 w568]
                          disable-tunnel: w559 -> [w566 w569]
                          disable-tunnel: [w563 w568] -> w558
                          disable-tunnel: [w562 w569] -> w557
                          frame Enabled {
                            w561 = FALSE ("Open Ser(t)")
                            w565 = u16 1 items=["MHz", "GHz"] ("Freq Units")
                            n253 = local read "RF_FREQ"() -> (w564:dbl)
                            n254 = call "Tetra_Set-Freq.vi"("COMPORT"=w566, "error in (no error)"=w567, "Freq"=w564, "Freq Units"=w565, "Open Ser(t)"=w561, "Close Ser(t)"=w561) -> ("comport"=w562:refnum<visa-resource-name>, "error out"=w563:errorcluster)  [unwired: 10 in, 2 out]
                          }
                          frame Disabled {
                          }
                        }
                      }
                    }
                    n255 = case shown="True" w538 {
                      tunnel: w527 -> [w582 w588]
                      tunnel: w526 -> [w583 w586]
                      tunnel: [w583 w592] -> w549
                      tunnel: [w582 w590] -> w550
                      tunnel: [i32[] [-1] ("atten(code)ary (ro)") _] -> _
                      tunnel: [w581 w584] -> w525
                      frame False {
                        n256 = global read "Tetra_Globals.vi" "Atten0"() -> (w581:dbl)
                      }
                      frame True {
                        n257 = global read "Tetra_Globals.vi" "RevC(t)"() -> (w589:bool)
                        n258 = local read "ADAR ATT"() -> (w591:dbl)
                        n259 = local read "adar_id"() -> (w587:i32)
                        n260 = call "Tetra_Atten.vi"("COMPORT"=w588, "RevC(T)"=w589, "error in (no error)"=w586, "TxAtten(num)"=w587, "Atten(dB)"=w591, "RO(t)"=TRUE) -> ("atten(value)"=w584:dbl, "comport"=w590:refnum<visa-resource-name>, "error out"=w592:errorcluster)  [unwired: 9 in, 2 out]
                      }
                    }
                    n261 = local read "RF_FREQ(t)"() -> (w540:bool)
                    n262 = local read "EXT_ATT(t)"() -> (w548:bool)
                    n263 = local read "use-psa(t)"() -> (w541:bool)
                    n264 = And(x=w548, y=w541) -> (x .and. y?=w547:bool)
                    n265 = And(x=w541, y=w540) -> (x .and. y?=w539:bool)
                    n266 = Or(x=w547, y=w539) -> (x .or. y?=w542:bool)
                    n267 = Or(x=w542, y=w533) -> (x .or. y?=w536:bool)
                    n268 = case shown="True" w536 {
                      tunnel: w550 -> [_ w579]
                      tunnel: w549 -> [w572 _]
                      tunnel: [w572 w578] -> w546
                      tunnel: [w571 w575] -> w524
                      tunnel: [w570 w574] -> w522
                      frame False {
                        n269 = global read "Tetra_Globals.vi" "txatten-sel"() -> (w570:i32)
                        n270 = global read "Tetra_Globals.vi" "Atten1-3"() -> (w571:dbl)
                      }
                      frame True {
                        n271 = global read "Tetra_Globals.vi" "RevC(t)"() -> (w576:bool)
                        n272 = local read "adar_id"() -> (w574:i32)
                        n273 = local read "EXT_ATT"() -> (w577:dbl)
                        n274 = call "Tetra_Atten.vi"("COMPORT"=w579, "RevC(T)"=w576, "TxAtten(num)"=w574, "Atten(dB)"=w577, "RO(t)"=TRUE) -> ("atten(value)"=w575:dbl, "error out"=w578:errorcluster)  [unwired: 10 in, 3 out]
                      }
                    }
                  }
                }
                "adar-att(val)" <- w443
                "ext-atten(val)" <- w444
                "txatten-sel" <- w437
                "atten(code)ary (ro)" <- w445
                "filt(num)" <- w442
                n275 = global write "Tetra_Globals.vi" "txatten-sel"(w437) -> ()
                n276 = global write "Tetra_Globals.vi" "Atten0"(w443) -> ()
                n277 = global write "Tetra_Globals.vi" "Atten1-3"(w444) -> ()
                n278 = global write "Tetra_Globals.vi" "atten(code)ary (ro)"(w445) -> ()
                n279 = global write "Tetra_Globals.vi" "TX_FILTER"(w442) -> ()
              }
            }
          }
          frame #11 {
            n280 = local read "do cmd?(f)"() -> (w606:bool)
            n281 = local read "comport"() -> (w605:refnum<visa-resource-name>)
            n282 = case shown="False" w606 {
              tunnel: w605 -> [w612 _]
              tunnel: w604 -> [w611 w615]
              tunnel: [w610 w615] -> w603
              frame False {
                n283 = local read "cmd;"() -> (w613:string)
                n284 = call "SerRW-Array.vi"("COMPORT"=w612, "error in (no error)"=w611, "Command ( ; seperation)"=w613) -> ("error out"=w610:errorcluster)  [unwired: 6 in, 6 out]
              }
              frame True {
                n285 = local write "cmd;"("-1" ("cmd;")) -> ()
              }
            }
            n286 = call <vilib>:"High Resolution Relative Seconds.vi"() -> ("relative seconds"=w609:dbl)
            n287 = Subtract(x=w609, y=w608) -> (x-y=→"x-y":dbl)
          }
          frame #12 {
            n288 = flat-sequence {
              tunnel: [w626] -> w617
              tunnel: w616 -> [w625]
              frame #0 {
                # "Get the DC Currents from Power Sup"
                n289 = local read "V_SUPPLY(t)"() -> (w623:bool)
                n290 = local read "TEMP(t)"() -> (w622:bool)
                n291 = local read "MEAS_PS"() -> (w624:bool)
                n292 = Or(x=w623, y=w622) -> (x .or. y?=w621:bool)
                n293 = local read "TX_PORT(t)"() -> (w618:bool)
                n294 = Or(x=w621, y=w624) -> (x .or. y?=w619:bool)
                n295 = Or(x=w618, y=w619) -> (x .or. y?=w620:bool)
                n296 = case shown="True" w620 {
                  tunnel: [dbl[] [-1.0, -1.0] w633] -> w627
                  tunnel: [w629 w636] -> w626
                  tunnel: w625 -> [w629 w637]
                  frame False {
                  }
                  frame True {
                    w640 = 0 items=["Current", "Voltage"] ("Measurement Type (1: Voltage)")
                    w639 = "PS1"  # SEL_PS
                    n297 = global read "Station References Global.vi" "PS1"() -> (w638:refnum<visa-resource-name>)
                    n298 = call "PS_MEASURE_V-I_Ary.vi"("VISA resource name"=w638, "SEL_PS"=w639, "error in (no error)"=w637, "Array 2"=bool[] [TRUE, FALSE, FALSE, FALSE], "Measurement Type (1: Voltage)"=w640) -> ("Array"=w634:dbl[], "error out"=w636:errorcluster)  [unwired: 8 in, 1 out]
                    n299 = local read "V_SUPPLY"() -> (w632:dbl)
                    n300 = Index Array(array=w634) -> (element=w630:dbl)  [unwired: 1 in]
                    n301 = Multiply(x=w630, y=w632) -> (x*y=w631:dbl)
                    n302 = Build Array(w630, w631) -> (w633:dbl[])
                  }
                }
                "ps_meas(i)(w)" <- w627
              }
            }
          }
          frame #13 {
          }
          frame #14 {
            n303 = flat-sequence {
              tunnel: w647 -> [w650]
              tunnel: [w648] -> w646
              tunnel: w646 -> [w665]
              tunnel: [w663] -> w645
              tunnel: w645 -> [w677]
              tunnel: [w676] -> w644
              tunnel: w644 -> [w682]
              tunnel: [w681] -> w643
              tunnel: w643 -> [w762]
              tunnel: [w741] -> w642
              frame #0 {
                # "Set The REF power"
                n304 = local read "REF_PWR(t)"() -> (w649:bool)
                n305 = case shown="True" w649 {
                  tunnel: w650 -> [w651 w661]
                  tunnel: [w651 w662] -> w648
                  frame False {
                  }
                  frame True {
                    (unwired) FALSE ("RO(T)")
                    w659 = 1 ("CH")
                    n306 = local read "REF_POW"() -> (w658:dbl)
                    n307 = Less?(x=w658, y=0.0) -> (x < y?=w656:bool)
                    n308 = global read "Station References Global.vi" "PNA"() -> (w660:refnum<visa-resource-name>)
                    n309 = Select(t=20.0, s=w656, f=0.0 ("Attenuation (0 dB)")) -> (s? t:f=w652:dbl)
                    "pna-att" <- w652
                    n310 = call "Configure Power.vi"("VISA resource name"=w660, "Enable Auto Attenuation (T: Enable)"=FALSE, "Channel (1)"=w659, "Port (1)"=w659, "Attenuation (0 dB)"=w652, "error in (no error)"=w661, "Power Level (0 dBm)"=w658) -> ("error out"=w662:errorcluster)  [unwired: 7 in, 1 out]
                  }
                }
              }
              frame #1 {
                # "Set The REF Fixed Freq"
                n311 = local read "RF_FREQ(t)"() -> (w664:bool)
                n312 = case shown="True" w664 {
                  tunnel: w665 -> [w666 w674]
                  tunnel: [w666 w670] -> w663
                  frame False {
                  }
                  frame True {
                    w667 = 0 items=["Normal", "SMC"] ("MODE")
                    w668 = i64 1000000000 items=["GHz"=1000000000, "MHZ"=1000000] ("Units")
                    n313 = global read "Station References Global.vi" "PNA"() -> (w675:refnum<visa-resource-name>)
                    n314 = local read "f_ref"() -> (w671:dbl)
                    n315 = call "PNA-L_SET-CWFREQ.vi"("Session In"=w675, "error in"=w674, "MODE"=w667, "FREQ"=w671, "Units"=w668, "RO(T)"=FALSE, "CH"=1, "Source"=1) -> ("error out"=w670:errorcluster)  [unwired: 9 in, 2 out]
                  }
                }
              }
              frame #2 {
                w679 = 3 items=["HOLD", "CONT", "GROUP", "SINGLE"]  # Mode
                w678 = 1  # Channel
                # "Take the Sweep with The PNA"
                n316 = global read "Station References Global.vi" "PNA"() -> (w680:refnum<visa-resource-name>)
                n317 = call "PNA_SWEEP MODE.vi"("Mode"=w679, "Channel"=w678, "error in (no error)"=w677, "VISA resource name"=w680) -> ("error out"=w676:errorcluster)  [unwired: 6 in, 1 out]
              }
              frame #3 {
                n318 = local read "MEAS_S11"() -> (w683:bool)
                n319 = case shown="True" w683 {
                  tunnel: w682 -> [w686 w689]
                  tunnel: [w686 w688] -> w681
                  tunnel: [-99.0 w690] -> w684
                  frame False {
                  }
                  frame True {
                    n320 = case shown="False" "GetS11FromFile?(t)" {
                      tunnel: [w710 w730] -> w690
                      tunnel: w689 -> [w702 w731]
                      tunnel: [w696 w727] -> w688
                      frame False {
                        w692 = 3 items=["HOLD", "CONT", "GROUP", "SINGLE"] ("Mode")
                        w699 = FALSE ("Enable Auto Attenuation (T: Enable)")
                        w693 = 3 items=["HOLD", "CONT", "GROUP", "SINGLE"] ("Mode")
                        w700 = 0.0 ("Power Level (0 dBm)")
                        w695 = 1  # Channel (1)
                        # "Meas S11 on the PNA"
                        # "Set to REF for Power"
                        # "Set to 0 for S11"
                        n321 = global read "Station References Global.vi" "PNA"() -> (w706:refnum<visa-resource-name>)
                        n322 = call "Configure Power.vi"("VISA resource name"=w706, "Enable Auto Attenuation (T: Enable)"=w699, "Channel (1)"=w695, "Port (1)"=w695, "Attenuation (0 dB)"=w700, "error in (no error)"=w702, "Power Level (0 dBm)"=w700) -> ("VISA resource name out"=w708:refnum<visa-resource-name>, "error out"=w709:errorcluster)  [unwired: 7 in]
                        n323 = call "PNA_SWEEP MODE.vi"("Mode"=w693, "Channel"=w695, "error in (no error)"=w709, "VISA resource name"=w708) -> ("error out"=w701:errorcluster, "VISA resource name out"=w707:refnum<visa-resource-name>)  [unwired: 6 in]
                        n324 = for {
                          N: 2 -> [_]
                          tunnel: [w714] -> w710
                          tunnel: w695 -> [w715]
                          shift-right: [w717] -> w704
                          shift-left: w707 -> [w719]
                          shift-right: [w718] -> w705
                          shift-left: w701 -> [w716]
                          stop <- w712 stop-if-true
                          n325 = local read "s11_hsl"() -> (w711:dbl)
                          n326 = local read "s11_lsl"() -> (w713:dbl)
                          n327 = call "Select Measurement.vi"("error in (no error)"=w716, "Measurement Name (CH1_S11_1)"="CH1_S11_1", "Channel (1)"=w715, "VISA resource name"=w719) -> ("error out"=w721:errorcluster, "VISA resource name out"=w722:refnum<visa-resource-name>)  [unwired: 6 in]
                          n328 = call "PNA-L_MKR_RageATE.vi"("VISA resource name"=w722, "Channel (1)"=w715, "Trace (1)"=w715, "Marker (1)"=w715, "error in (no error)"=w721) -> ("VISA resource name out"=w717:refnum<visa-resource-name>, "Y Real Value"=w714:dbl, "error out"=w718:errorcluster)  [unwired: 6 in, 2 out]
                          n329 = In Range and Coerce(upper limit=w711, x=w714, lower limit=w713) -> (In Range?=w712:bool)  [unwired: 1 out]
                        }
                        n330 = local read "pna-att"() -> (w694:dbl)
                        n331 = local read "REF_POW"() -> (w703:dbl)
                        n332 = call "Configure Power.vi"("VISA resource name"=w704, "Enable Auto Attenuation (T: Enable)"=w699, "Channel (1)"=w695, "Port (1)"=w695, "Attenuation (0 dB)"=w694, "error in (no error)"=w705, "Power Level (0 dBm)"=w703) -> ("VISA resource name out"=w698:refnum<visa-resource-name>, "error out"=w697:errorcluster)  [unwired: 7 in]
                        n333 = call "PNA_SWEEP MODE.vi"("Mode"=w692, "Channel"=w695, "error in (no error)"=w697, "VISA resource name"=w698) -> ("error out"=w696:errorcluster)  [unwired: 6 in, 1 out]
                      }
                      frame True {
                        n334 = global read "Tetra_Globals.vi" "s11_path"() -> (w723:path)
                        n335 = local read "f_ref"() -> (w725:dbl)
                        n336 = call "GetCalData.vi"("Open new file T"=TRUE, "error in (no error)"=w731, "RF Freq (MHz)"=w725, "cal file path (dialog if empty)"=w723) -> ("error out"=w728:errorcluster, "Ampl Out"=w730:dbl, "Coerced(T)"=w724:bool)  [unwired: 2 in, 3 out]
                        n337 = case shown="True" w724 {
                          tunnel: w724 -> [_ w740]
                          tunnel: w728 -> [w732 w739]
                          tunnel: [w732 w738] -> w727
                          tunnel: [FALSE w734] -> w726
                          frame False {
                          }
                          frame True {
                            n338 = call "TimeOutPopUp.vi"("Enable"=w740, "error in (no error)"=w739, "Timeout(s)"=10, "Input Message"="There is no S11 Frequency Match. Check the Calibration and Frequency List.\nAlso Check the Frequency Units Match.") -> ("OK"=w735:bool, "error out"=w738:errorcluster)  [unwired: 13 in, 1 out]
                            n339 = Not(x=w735) -> (.not. x?=w734:bool)
                          }
                        }
                        n340 = global write "Sequence Globals.vi" "Stop Testing"(w726) -> ()
                        n341 = local write "STOP(T)"(w726) -> ()
                      }
                    }
                  }
                }
                "s11" <- w684
              }
              frame #4 {
                n342 = global read "Station References Global.vi" "Spectrum Analyzer Present?"() -> (w760:bool)
                n343 = case shown="True" w760 {
                  tunnel: w762 -> [w818 w825]
                  tunnel: [dbl[] [-1.0, -1.0] ("Mark Values") w823] -> w761
                  tunnel: [w818 w824] -> w759
                  tunnel: [w817 w822] -> w753
                  tunnel: [w817 w821] -> w749
                  frame False {
                    w817 = -1.0 ("Ampl_corr")
                  }
                  frame True {
                    n344 = for {
                      N: 5 -> [w837]
                      tunnel: [w833] -> w823
                      tunnel: [w834] -> w822
                      tunnel: [w826] -> w821
                      shift-right: [w828] -> w824
                      shift-left: w825 -> [w838]
                      i -> [w836]
                      stop <- w827 stop-if-true
                      n345 = flat-sequence {
                        tunnel: w838 -> [w842]
                        tunnel: w837 -> [w841]
                        tunnel: w836 -> [w839]
                        tunnel: [w843] -> w835
                        tunnel: [w840] -> w832
                        tunnel: w835 -> [w872]
                        tunnel: [w874] -> w834
                        tunnel: [w873] -> w833
                        tunnel: w832 -> [w871]
                        tunnel: [w871] -> w831
                        tunnel: [w870] -> w830
                        tunnel: [w869] -> w829
                        tunnel: [w868] -> w826
                        tunnel: w831 -> [w898]
                        tunnel: w830 -> [w897]
                        tunnel: w829 -> [w896]
                        tunnel: [w896] -> w828
                        tunnel: [w895] -> w827
                        frame #0 {
                          n346 = case shown="1.." w839 {
                            tunnel: w842 -> [w845 w863]
                            tunnel: [w845 w867] -> w843
                            tunnel: [TRUE w859] -> w840
                            tunnel: w841 -> [_ w851]
                            tunnel: w839 -> [_ w860]
                            frame 0, Default {
                            }
                            frame 1.. {
                              w857 = i64 1000000000 items=["GHz"=1000000000, "MHZ"=1000000] ("Units")
                              w848 = FALSE ("RO(T)")
                              w853 = 1 ("Source")
                              w854 = 3 items=["HOLD", "CONT", "GROUP", "SINGLE"] ("Mode")
                              w852 = 0 items=["Normal", "SMC"] ("MODE")
                              # "workaround for freq set issue on N5232A\nSet freq to other, then back to original"
                              n347 = local read "f_ref"() -> (w847:dbl)
                              n348 = Increment(x=w860) -> (x+1=w850:i32)
                              n349 = call <vilib>:"Clear Errors.vi"("error in (no error)"=w863) -> ("error out"=w846:errorcluster)  [unwired: 5 in, 1 out]
                              n350 = Add(x=w847, y=0.1) -> (x+y=w862:dbl)
                              n351 = Equal?(x=w851, y=w850) -> (x = y?=w859:bool)
                              n352 = global read "Station References Global.vi" "PNA"() -> (w864:refnum<visa-resource-name>)
                              n353 = call "PNA-L_SET-CWFREQ.vi"("Session In"=w864, "error in"=w846, "MODE"=w852, "FREQ"=w862, "Units"=w857, "RO(T)"=w848, "CH"=w853, "Source"=w853) -> ("Session Out"=w855:refnum<visa-resource-name>, "error out"=w856:errorcluster)  [unwired: 9 in, 1 out]
                              n354 = call "PNA_SWEEP MODE.vi"("Mode"=w854, "Channel"=w853, "error in (no error)"=w856, "VISA resource name"=w855) -> ("error out"=w858:errorcluster, "VISA resource name out"=w849:refnum<visa-resource-name>)  [unwired: 6 in]
                              n355 = call "PNA-L_SET-CWFREQ.vi"("Session In"=w849, "error in"=w858, "MODE"=w852, "FREQ"=w847, "Units"=w857, "RO(T)"=w848, "CH"=w853, "Source"=w853) -> ("Session Out"=w865:refnum<visa-resource-name>, "error out"=w866:errorcluster)  [unwired: 9 in, 1 out]
                              n356 = call "PNA_SWEEP MODE.vi"("Mode"=w854, "Channel"=w853, "error in (no error)"=w866, "VISA resource name"=w865) -> ("error out"=w867:errorcluster)  [unwired: 6 in, 1 out]
                            }
                          }
                          "txp_#ofretries" <- w839
                        }
                        frame #1 {
                          w880 = 1 items=["Clear Write", "Average", "Maximum Hold", "Minimum Hold"] ("Trace Type (0: Clear Write)")
                          w882 = i64 1000000000 items=["Hz"=1, "KHz"=1000, "MHz"=1000000, "GHz"=1000000000] ("Units")
                          w876 = u16 2 items=["Hz", "MHz", "GHz"] ("Freq Units")
                          n357 = local read "bypass ESA Freq Set(t)"() -> (w891:bool)
                          n358 = local read "RF_FREQ"() -> (w885:dbl)
                          n359 = global read "Station References Global.vi" "Spectrum Analyzer"() -> (w883:refnum<visa-resource-name>)
                          n360 = call "SA_SET_CF.vi"("Send OPC? (T)"=TRUE, "READ ONLY (T)"=w891, "error in"=w872, "Freq Units"=w876, "SET CF ()"=w885, "Session In"=w883) -> ("error out"=w888:errorcluster, "Session Out"=w887:refnum<visa-resource-name>)  [unwired: 3 in, 1 out]
                          n361 = local read "out_cal_ampl"() -> (w889:dbl)
                          n362 = local read "AVG"() -> (w884:i32)
                          n363 = call "SA_AVG.vi"("Session In"=w887, "AVG Count"=w884, "error in"=w888, "Trace Type (0: Clear Write)"=w880, "AVG Restart (T)"=TRUE, "Send OPC? (T)"=TRUE ("AVG Restart (T)")) -> ("Session Out"=w886:refnum<visa-resource-name>, "error out"=w892:errorcluster)  [unwired: 8 in]
                          n364 = local read "fsl_corr_dB"() -> (w890:dbl)
                          n365 = call "SA_GET_MARKER.vi"("Units"=w882, "offset"=w889, "Set MKR Freq ()"=w885, "Use PK Search (T)"=TRUE, "error in"=w892, "Session In"=w886) -> ("error out"=w869:errorcluster, "Ampl_corr"=w874:dbl, "Mark Values"=w873:dbl[])  [unwired: 2 in, 1 out]
                          n366 = Index Array(array=w873, index=1) -> (element=w870:dbl)
                          n367 = Add(x=w874, y=w890) -> (x+y=w868:dbl)
                        }
                        frame #2 {
                          # "Anti Glitch\nretry if not\nwithin"
                          n368 = In Range and Coerce(upper limit=-0.1, x=w897, lower limit=-105.0) -> (In Range?=w895:bool)  [unwired: 1 out]
                          n369 = Not(x=w895) -> (.not. x?=w894:bool)
                          n370 = And(x=w894, y=w898) -> (x .and. y?=→"AntiGlitch?(t)":bool)
                        }
                      }
                    }
                  }
                }
                "exa_mkr" <- w761
                "Ampl_corr" <- w753
                "fsl_ampl_corr" <- w749
                n371 = global read "Station References Global.vi" "Spectrum Analyzer Present?"() -> (w756:bool)
                n372 = local read "h2(t)"() -> (w755:bool)
                n373 = And(x=w756, y=w755) -> (x .and. y?=w757:bool)
                n374 = case shown="True" w757 {
                  tunnel: w759 -> [w791 w815]
                  tunnel: [dbl[] [-1.0, -1.0] ("Mark Values") w802] -> w758
                  tunnel: [w791 w804] -> w747
                  tunnel: [w790 w801] -> w754
                  tunnel: [w790 w795] -> w752
                  tunnel: [w790 w795] -> w748
                  frame False {
                    w790 = -1.0
                    n375 = local write "h2_cal_ampl"(w790) -> ()
                    n376 = local write "h2_cal freq"(w790) -> ()
                  }
                  frame True {
                    w794 = i64 1000000000 items=["Hz"=1, "KHz"=1000, "MHz"=1000000, "GHz"=1000000000] ("Units")
                    w803 = u16 2 items=["Hz", "MHz", "GHz"] ("Freq Units")
                    w811 = 1 items=["Clear Write", "Average", "Maximum Hold", "Minimum Hold"] ("Trace Type (0: Clear Write)")
                    n377 = global read "Station References Global.vi" "Spectrum Analyzer"() -> (w816:refnum<visa-resource-name>)
                    n378 = local read "bypass ESA Freq Set(t)"() -> (w799:bool)
                    n379 = local read "H2_FREQ"() -> (w806:dbl)
                    n380 = call "SA_SET_CF.vi"("Send OPC? (T)"=TRUE, "READ ONLY (T)"=w799, "error in"=w815, "Freq Units"=w803, "SET CF ()"=w806, "Session In"=w816) -> ("error out"=w812:errorcluster, "Session Out"=w813:refnum<visa-resource-name>)  [unwired: 3 in, 1 out]
                    n381 = local read "AVG_HARM"() -> (w809:i32)
                    n382 = local read "h2_cal_ampl"() -> (w800:dbl)
                    n383 = call "SA_AVG.vi"("Session In"=w813, "AVG Count"=w809, "error in"=w812, "Trace Type (0: Clear Write)"=w811, "AVG Restart (T)"=TRUE, "Send OPC? (T)"=TRUE ("AVG Restart (T)")) -> ("Session Out"=w807:refnum<visa-resource-name>, "error out"=w808:errorcluster)  [unwired: 8 in]
                    n384 = local read "h2_fsl_corr"() -> (w798:dbl)
                    n385 = call "SA_GET_MARKER.vi"("Units"=w794, "offset"=w800, "Set MKR Freq ()"=w806, "Use PK Search (T)"=FALSE, "error in"=w808, "Session In"=w807) -> ("error out"=w804:errorcluster, "Ampl_corr"=w797:dbl, "Mark Values"=w802:dbl[])  [unwired: 2 in, 1 out]
                    n386 = local read "fsl_ampl_corr"() -> (w796:dbl)
                    n387 = Add(x=w797, y=w798) -> (x+y=w795:dbl)
                    n388 = Subtract(x=w795, y=w796) -> (x-y=w801:dbl)
                  }
                }
                "h2_mkr" <- w758
                "h2_dbc" <- w754
                "h2_corr" <- w752
                "h2_fsl_ampl_corr" <- w748
                n389 = global read "Station References Global.vi" "Spectrum Analyzer Present?"() -> (w750:bool)
                n390 = local read "hx(t)"() -> (w751:bool)
                n391 = And(x=w750, y=w751) -> (x .and. y?=w746:bool)
                n392 = case shown="True" w746 {
                  tunnel: w747 -> [w764 w788]
                  tunnel: [dbl[] [-1.0, -1.0] ("Mark Values") w775] -> w745
                  tunnel: [w764 w777] -> w741
                  tunnel: [w763 w774] -> w744
                  tunnel: [w763 w769] -> w743
                  tunnel: [w763 w769] -> w742
                  frame False {
                    w763 = -1.0
                    n393 = local write "hx_cal_ampl"(w763) -> ()
                    n394 = local write "hx_cal freq"(w763) -> ()
                  }
                  frame True {
                    (unwired) FALSE ("AVG Restart (T)")
                    w767 = i64 1000000000 items=["Hz"=1, "KHz"=1000, "MHz"=1000000, "GHz"=1000000000] ("Units")
                    w776 = u16 2 items=["Hz", "MHz", "GHz"] ("Freq Units")
                    w784 = 1 items=["Clear Write", "Average", "Maximum Hold", "Minimum Hold"] ("Trace Type (0: Clear Write)")
                    n395 = global read "Station References Global.vi" "Spectrum Analyzer"() -> (w789:refnum<visa-resource-name>)
                    n396 = local read "bypass ESA Freq Set(t)"() -> (w772:bool)
                    n397 = local read "Hx_FREQ"() -> (w779:dbl)
                    n398 = call "SA_SET_CF.vi"("Send OPC? (T)"=TRUE, "READ ONLY (T)"=w772, "error in"=w788, "Freq Units"=w776, "SET CF ()"=w779, "Session In"=w789) -> ("error out"=w785:errorcluster, "Session Out"=w786:refnum<visa-resource-name>)  [unwired: 3 in, 1 out]
                    n399 = local read "AVG_HARM"() -> (w782:i32)
                    n400 = local read "hx_cal_ampl"() -> (w773:dbl)
                    n401 = call "SA_AVG.vi"("Session In"=w786, "AVG Count"=w782, "error in"=w785, "Trace Type (0: Clear Write)"=w784, "AVG Restart (T)"=TRUE, "Send OPC? (T)"=TRUE ("AVG Restart (T)")) -> ("Session Out"=w780:refnum<visa-resource-name>, "error out"=w781:errorcluster)  [unwired: 8 in]
                    n402 = local read "hx_fsl_corr"() -> (w771:dbl)
                    n403 = call "SA_GET_MARKER.vi"("Units"=w767, "offset"=w773, "Set MKR Freq ()"=w779, "Use PK Search (T)"=FALSE, "error in"=w781, "Session In"=w780) -> ("error out"=w777:errorcluster, "Ampl_corr"=w770:dbl, "Mark Values"=w775:dbl[])  [unwired: 2 in, 1 out]
                    n404 = local read "fsl_ampl_corr"() -> (w768:dbl)
                    n405 = Add(x=w770, y=w771) -> (x+y=w769:dbl)
                    n406 = Subtract(x=w769, y=w768) -> (x-y=w774:dbl)
                  }
                }
                "hx_dbc" <- w744
                "hx_mkr" <- w745
                "hx_corr" <- w743
                "hx_fsl_ampl_corr" <- w742
              }
            }
          }
          frame #15 {
            # "Get the chip stuff..."
            n407 = flat-sequence {
              tunnel: w903 -> [w908]
              tunnel: [w907] -> w905
              tunnel: w905 -> [w927]
              tunnel: [w928] -> w904
              tunnel: w904 -> [w960]
              tunnel: [w962] -> w902
              tunnel: [w982] -> w901
              tunnel: w902 -> [w983]
              frame #0 {
                # "Get the Power detector"
                n408 = local read "GET_DETECT"() -> (w906:bool)
                n409 = case shown="True" w906 {
                  tunnel: [-99.0 w917] -> w909
                  tunnel: w908 -> [w910 w915]
                  tunnel: [w910 w916] -> w907
                  frame False {
                  }
                  frame True {
                    n410 = global read "Tetra_Globals.vi" "RevC(t)"() -> (w912:bool)
                    n411 = local read "comport"() -> (w913:refnum<visa-resource-name>)
                    n412 = local read "TX_PORT"() -> (w914:i32)
                    n413 = call "TX-ADAR-DETECT(LC).vi"("COMPORT"=w913, "RevC(t)"=w912, "error in (no error)"=w915, "Ant_Sel"=w914) -> ("adc read"=w917:dbl, "error out"=w916:errorcluster)  [unwired: 8 in, 2 out]
                  }
                }
                "detect" <- w909
              }
              frame #1 {
                n414 = local read "MEAS_DCMON"() -> (w923:bool)
                n415 = local read "TEMP(t)"() -> (w924:bool)
                n416 = local read "MEAS_DCMON"() -> (w925:bool)
                n417 = local read "V_SUPPLY(t)"() -> (w921:bool)
                n418 = local read "TX_PORT(t)"() -> (w918:bool)
                n419 = Or(x=w924, y=w923) -> (x .or. y?=w922:bool)
                n420 = Or(x=w922, y=w925) -> (x .or. y?=w926:bool)
                n421 = Or(x=w918, y=w921) -> (x .or. y?=w919:bool)
                n422 = Or(x=w926, y=w919) -> (x .or. y?=w920:bool)
                n423 = case shown="False" w920 {
                  tunnel: [w938 w953] -> w929
                  tunnel: [w938 w952] -> w930
                  tunnel: [w937 w951] -> w928
                  tunnel: [w939 w950] -> w931
                  tunnel: w927 -> [w937 w945]
                  frame False {
                    n424 = global read "Tetra_Globals.vi" "RevC(t)"() -> (w933:bool)
                    n425 = Select(t=11, s=w933, f=11) -> (s? t:f=w936:i32)
                    n426 = for {
                      N: 6 -> [_]
                      tunnel: [-1.0] -> w938 mode=indexing
                    }
                    n427 = for {
                      N: w936 -> [_]
                      tunnel: [-1.0] -> w939 mode=indexing
                    }
                  }
                  frame True {
                    n428 = local read "comport"() -> (w944:refnum<visa-resource-name>)
                    n429 = call "Tetra_Read UCD.vi"("COMPORT"=w944, "error in (no error)"=w945) -> ("rdv"=w950:dbl[], "comport"=w948:refnum<visa-resource-name>, "error out"=w949:errorcluster)  [unwired: 11 in]
                    n430 = global read "Tetra_Globals.vi" "RevC(t)"() -> (w942:bool)
                    n431 = call "Time Delay"("error in (no error)"=w949, "Delay Time (s)"=0.01) -> ("error out"=w947:errorcluster)  [unwired: 9 in]
                    n432 = call "Tetra_Read Imon.vi"("COMPORT"=w948, "rev_c(t)"=w942, "error in (no error)"=w947, "Meas_Limits"=FALSE) -> ("rdiv(i)"=w953:dbl[], "rdiv(v)"=w952:dbl[], "error out"=w951:errorcluster)  [unwired: 10 in, 3 out]
                  }
                }
                "rdiv(i)" <- w929
                "rdiv(v)" <- w930
                "rdv" <- w931
              }
              frame #2 {
                n433 = local read "TX_PORT(t)"() -> (w954:bool)
                n434 = local read "CHIP_TEMP(t)"() -> (w959:bool)
                n435 = First Call?() -> (First Call?: T/F=w956:bool)
                n436 = Or(x=w954, y=w956) -> (x .or. y?=w955:bool)
                n437 = Or(x=w959, y=w955) -> (x .or. y?=w957:bool)
                n438 = case shown="True" w957 {
                  tunnel: [w964 w967] -> w962
                  tunnel: [dbl[] [-99.0, -99.0, -99.0, -99.0, -99.0, -99.0] ("Deg") w968] -> w958
                  tunnel: w960 -> [w964 w976]
                  tunnel: ["-1" ("temp 0x") w975] -> w961
                  frame False {
                  }
                  frame True {
                    n439 = global read "Tetra_Globals.vi" "RevC(t)"() -> (w966:bool)
                    n440 = local read "comport"() -> (w974:refnum<visa-resource-name>)
                    n441 = call "TX-ADAR-TEMP.vi"("COMPORT"=w974, "RevC(t)"=w966, "error in (no error)"=w976) -> ("temp 0x"=w975:string, "comport"=w973:refnum<visa-resource-name>, "temp(c)"=w970:dbl, "error out"=w972:errorcluster)  [unwired: 9 in]
                    n442 = call "ReadTempSense.vi"("COMPORT"=w973, "error in (no error)"=w972) -> ("temp(c)"=w971:dbl[], "error out"=w967:errorcluster)  [unwired: 10 in, 2 out]
                    n443 = Insert Into Array(array=w971, index=0, new element=w970) -> (w968:dbl[])
                  }
                }
                "temp_data" <- w958
                "temp 0x" <- w961
              }
              frame #3 {
                n444 = local read "TxFiltRead"() -> (w977:bool)
                n445 = local read "MODE"() -> (w978:bool)
                n446 = Or(x=w978, y=w977) -> (x .or. y?=w979:bool)
                n447 = case shown="True" w979 {
                  tunnel: w983 -> [w985 w999]
                  tunnel: [w985 w996] -> w982
                  tunnel: [w984 w993] -> w981
                  tunnel: [w984 w989] -> w980
                  frame False {
                    w984 = -1 ("bpf")
                  }
                  frame True {
                    w991 = 1 items=["RX", "TX"] ("RX/TX")
                    w1001 = 1 items=["RX", "TX"] ("RX/TX")
                    n448 = local read "comport"() -> (w998:refnum<visa-resource-name>)
                    n449 = global read "Tetra_Globals.vi" "RevC(t)"() -> (w988:bool)
                    n450 = local read "adar_id"() -> (w987:i32)
                    n451 = call "Tetra_Filt.vi"("COMPORT"=w998, "ADAR-ID"=w987, "Rev-C(T)"=w988, "error in (no error)"=w999, "RO(t)"=TRUE, "RX/TX"=w1001) -> ("filt(num)"=w989:i32, "comport"=w1003:refnum<visa-resource-name>, "error out"=w1002:errorcluster)  [unwired: 11 in]
                    n452 = local read "TX_PORT"() -> (w986:i32)
                    n453 = call "Tetra_Atten.vi"("COMPORT"=w1003, "RevC(T)"=w988, "error in (no error)"=w1002, "TxAtten(num)"=w987, "RO(t)"=TRUE) -> ("comport"=w994:refnum<visa-resource-name>, "atten(code)ary (ro)"=w997:i32[], "error out"=w995:errorcluster)  [unwired: 10 in, 2 out]
                    n454 = global write "Tetra_Globals.vi" "atten(code)ary (ro)"(w997) -> ()
                    n455 = local write "atten(code)ary (ro)"(w997) -> ()
                    n456 = call "Tetra_BPF.vi"("COMPORT"=w994, "Rev-C(t)"=w988, "ant-port"=w986, "error in (no error)"=w995, "RO(t)"=TRUE, "RX/TX"=w991) -> ("bpf"=w993:i32, "error out"=w996:errorcluster)  [unwired: 11 in, 1 out]
                  }
                }
                "bpf" <- w981
                n457 = local write "filt(num)"(w980) -> ()
                n458 = global write "Tetra_Globals.vi" "TX_FILTER"(w980) -> ()
              }
            }
          }
          frame #16 {
          }
          frame #17 {
            n459 = flat-sequence {
              tunnel: [w1016] -> w1006
              tunnel: w1005 -> [w1011]
              frame #0 {
                n460 = local read "PLATE_TEMP(t)"() -> (w1014:bool)
                n461 = local read "TX_PORT(t)"() -> (w1007:bool)
                n462 = global read "Station References Global.vi" "Oven Present?"() -> (w1012:bool)
                n463 = First Call?() -> (First Call?: T/F=w1009:bool)
                n464 = Or(x=w1014, y=w1009) -> (x .or. y?=w1010:bool)
                n465 = Or(x=w1007, y=w1010) -> (x .or. y?=w1008:bool)
                n466 = And(x=w1008, y=w1012) -> (x .and. y?=w1013:bool)
                n467 = case shown="False" w1013 {
                  tunnel: [w1018 w1022] -> w1016
                  tunnel: [sgl[] [-99.0, -99.0] w1020] -> w1015
                  tunnel: w1011 -> [w1018 w1021]
                  frame False {
                  }
                  frame True {
                    n468 = for {
                      N: 3 -> [_]
                      tunnel: [w1026] -> w1020
                      shift-right: [w1023] -> w1022
                      shift-left: w1021 -> [w1028]
                      stop <- w1023 continue-if-true
                      w1027 = u16 1 items=["SENSOR 1", "SENSOR 2"] ("Sensor")
                      w1033 = u16 0 items=["SENSOR 1", "SENSOR 2"] ("Sensor")
                      n469 = global read "Station References Global.vi" "Oven"() -> (w1035:refnum<visa-resource-name>)
                      n470 = call "PM9_TCP_READ-TEMP.vi"("VISA"=w1035, "error in (no error)"=w1028, "Sensor"=w1033, "Close tcp(t)"=FALSE) -> ("Value"=w1025:sgl, "visa out"=w1031:refnum<visa-resource-name>, "connection ID out"=w1030:refnum<k5>, "error out"=w1032:errorcluster)  [unwired: 8 in]
                      n471 = call "PM9_TCP_READ-TEMP.vi"("VISA"=w1031, "connection ID"=w1030, "error in (no error)"=w1032, "Sensor"=w1027, "Close tcp(t)"=TRUE) -> ("Value"=w1024:sgl, "error out"=w1023:errorcluster)  [unwired: 7 in, 2 out]
                      n472 = Build Array(w1025, w1024) -> (w1026:sgl[])
                    }
                  }
                }
                "plate_temp" <- w1015
              }
            }
          }
          frame #18 {
            n473 = flat-sequence {
              tunnel: [w1038] -> w1036
              frame #0 {
                w1039 = TRUE ("Close Serial")
                n474 = local read "ess_error"() -> (w1044:errorcluster)
                n475 = global read "Station References Global.vi" "Gantry"() -> (w1042:refnum<visa-resource-name>)
                n476 = local read "FH_NOT(T)"() -> (w1041:bool)
                n477 = call "WAM_ESS.vi"("VISA resource name"=w1042, "error in (no error)"=w1044, "Open Serial"=w1039, "Test Running (T)"=w1039, "Close Serial"=w1039) -> ("FH_NOT(T)"=w1040:bool, "VISA resource name out"=w1043:refnum<visa-resource-name>, "error out"=w1045:errorcluster)  [unwired: 7 in, 1 out]
                n478 = And(x=w1041, y=w1040) -> (x .and. y?=w1038:bool)
                "no_fault" <- w1038
                n479 = case shown="True" w1038 {
                  tunnel: w1043 -> [w1054 _]
                  tunnel: w1045 -> [w1053 w1060]
                  tunnel: [w1052 w1060] -> w1046
                  frame False {
                    w1050 = u16 1 items=["Disable Driver", "Enable Driver", "Read Driver Status"] ("Driver-Func")
                    w1051 = TRUE ("Close Serial")
                    n480 = call "Prompt User for Input"("error in (no error)"=w1053) -> ("OK"=w1049:bool, "error out"=w1048:errorcluster)  [unwired: 17 in]
                    n481 = case shown="False" w1049 {
                      selector: w1049 -> [w1056 _]
                      tunnel: w1048 -> [w1058 w1059]
                      tunnel: [w1057 w1059] -> w1047
                      frame False {
                        n482 = invoke class="VI" method="Abort VI"(error in=w1058) -> (error out=w1057:errorcluster)  [unwired: 2 in, 2 out]
                        n483 = Not(x=w1056) -> (.not. x?=w1055:bool)
                        n484 = local write "STOP(T)"(w1055) -> ()
                        n485 = global write "Sequence Globals.vi" "Stop Testing"(w1055) -> ()
                      }
                      frame True {
                      }
                    }
                    n486 = call "Gantry_Driver.vi"("VISA resource name"=w1054, "error in (no error)"=w1047, "Open Serial"=w1051, "Driver-Func"=w1050, "Close Serial"=w1051) -> ("error out"=w1052:errorcluster)  [unwired: 11 in, 3 out]
                  }
                  frame True {
                  }
                }
                n487 = local write "ess_error"(w1046) -> ()
              }
            }
          }
          frame #19 {
            n488 = local read "ser_rd"() -> (w1063:string)
            n489 = Empty String/Path?(string/path=w1063) -> (empty?=w1064:bool)
            n490 = case shown="True" w1064 {
              tunnel: [w1066 "null"] -> w1065
              tunnel: w1063 -> [w1076 _]
              tunnel: w1062 -> [w1075 w1077]
              tunnel: [w1074 w1077] -> w1061
              frame False {
                w1068 = TRUE ("replace all? (F)")
                n491 = local read "comport"() -> (w1073:refnum<visa-resource-name>)
                n492 = call <vilib>:"Space Constant.vi"() -> ("String"=w1069:string)
                n493 = call "SerRW-Array.vi"("COMPORT"=w1073, "error in (no error)"=w1075, "Command ( ; seperation)"=w1076) -> ("string"=w1067:string, "error out"=w1074:errorcluster)  [unwired: 6 in, 5 out]
                n494 = Search and Replace String(replace all?=w1068, input string=w1067, search string="\n", replace string=w1069) -> (result string=w1071:string)  [unwired: 4 in, 3 out]
                n495 = Search and Replace String(replace all?=w1068, input string=w1071, search string="\r", replace string=w1069) -> (result string=w1066:string)  [unwired: 4 in, 3 out]
              }
              frame True {
              }
            }
            "readback" <- w1065
          }
          frame #20 {
            # "Insert the output numeric array data"
            n496 = Unbundle By Name(w1079) -> ("status"=w1082:bool)
            n497 = local read "ps_meas(i)(w)"() -> (w1114:dbl[])
            n498 = local read "relative seconds"() -> (w1119:dbl)
            n499 = local read "atten(code)ary (ro)"() -> (w1095:i32[])
            n500 = global read "Sequence Globals.vi" "Current Iteration"() -> (w1118:i32)
            n501 = local read "horn_Ampl Out"() -> (w1083:dbl)
            n502 = local read "fsl_ampl_corr"() -> (w1086:dbl)
            n503 = local read "ext-atten(val)"() -> (w1112:dbl)
            n504 = local read "out_cal_ampl"() -> (w1103:dbl)
            n505 = call <vilib>:"High Resolution Relative Seconds.vi"() -> ("relative seconds"=w1120:dbl)
            "iteration time(s)" <- w1120
            n506 = local read "adar-att(val)"() -> (w1107:dbl)
            n507 = local read "h2_cal_ampl"() -> (w1098:dbl)
            n508 = local read "hx_cal_ampl"() -> (w1088:dbl)
            n509 = local read "out_cal freq"() -> (w1102:dbl)
            n510 = local read "plate_temp"() -> (w1109:sgl[])
            n511 = local read "temp_data"() -> (w1108:dbl[])
            n512 = local read "fsl_corr_dB"() -> (w1085:dbl)
            n513 = local read "h2_cal freq"() -> (w1097:dbl)
            n514 = local read "hx_cal freq"() -> (w1087:dbl)
            n515 = local read "Ampl_corr"() -> (w1101:dbl)
            n516 = local read "filt(num)"() -> (w1113:i32)
            n517 = local read "exa_mkr"() -> (w1111:dbl[])
            n518 = local read "h2_mkr"() -> (w1100:dbl[])
            n519 = local read "h2_corr"() -> (w1096:dbl)
            n520 = local read "h2_dbc"() -> (w1104:dbl)
            n521 = local read "hx_mkr"() -> (w1091:dbl[])
            n522 = local read "hx_corr"() -> (w1090:dbl)
            n523 = local read "hx_dbc"() -> (w1089:dbl)
            n524 = Subtract(x=w1120, y=w1119) -> (x-y=w1105:dbl)
            n525 = local read "rdiv(v)"() -> (w1116:dbl[])
            n526 = local read "fsl(dB)"() -> (w1084:dbl)
            n527 = local read "detect"() -> (w1110:dbl)
            n528 = local read "rdiv(i)"() -> (w1115:dbl[])
            n529 = local read "f_ref"() -> (w1099:dbl)
            n530 = local read "s11"() -> (w1106:dbl)
            n531 = local read "rdv"() -> (w1117:dbl[])
            n532 = local read "bpf"() -> (w1094:i32)
            n533 = Build Array (concatenate)(w1114, w1111, w1101, w1086, w1106, w1099, w1100, w1096, w1104, w1091, w1090, w1089, w1110, w1113, w1094, w1107, w1112, w1095, w1117, w1116, w1115, w1108, w1109, w1105, w1118, w1103, w1102, w1098, w1097, w1088, w1087, w1085, w1084, w1083) -> (w1093:dbl[])
            n534 = Not(x=w1082) -> (.not. x?=w1081:bool)
            n535 = for {
              tunnel: w1093 -> [w1126] mode=indexing
              tunnel: [w1124] -> w1092 mode=indexing
              tunnel: w1079 -> [w1122]
              tunnel: [w1121] -> w1080
              n536 = Format Into String(format string="%#.3f", initial string="", error in=w1122, w1126) -> (resulting string=w1124:string, error out=w1121:errorcluster)
            }
          }
        }
        n537 = Greater Than 0?(x=w53) -> (x > 0?=→"x > 0?":bool)
        n538 = And(x=w54, y=w50) -> (x .and. y?=w51:bool)
      }
    }
    frame #2 {
      n539 = flat-sequence {
        tunnel: [w1156] -> w1140
        tunnel: [w1153] -> w1138
        tunnel: w1140 -> [w1162]
        tunnel: [w1168] -> w1139
        tunnel: w1138 -> [w1163]
        tunnel: [w1163] -> w1137
        tunnel: [w1159] -> w1136
        tunnel: [w1158] -> w1134
        tunnel: [w1157] -> w1131
        tunnel: [w1288] -> w1141
        tunnel: w1139 -> [w1288]
        tunnel: w1137 -> [_]
        tunnel: w1136 -> [w1287]
        tunnel: [w1287] -> _
        tunnel: w1134 -> [w1285]
        tunnel: [w1283] -> _
        tunnel: [w1283] -> w1133
        tunnel: w1131 -> [w1282]
        frame #0 {
          # "Flag rows to report"
          n540 = local read "RF_FREQ"() -> (w1156:dbl)
          n541 = Equal?(x=w1156, y=dbl[] [25.0, 32.0, 40.0]) -> (x = y?=w1154:bool[])
          n542 = Or Array Elements(Boolean array=w1154) -> (logical OR=w1153:bool)
        }
        frame #1 {
          # "Store tx data for reatreival to calc  flatness\nThis is based on 2 \"bands\"of 20-25, 25-*40 GHz"
          n543 = Current VI's Path() -> (path=w1167:path)
          n544 = Strip Path(path=w1167) -> (stripped path=w1164:path)  [unwired: 1 out]
          n545 = local read "fsl_ampl_corr"() -> (w1170:dbl)
          n546 = Multiply(x=w1162, y=1000.0) -> (x*y=w1161:dbl)
          n547 = Build Array(w1162, w1170) -> (w1169:dbl[])
          n548 = Build Path(base path=w1164, name or relative path=path "txflat.txt" ("file path (dialog if empty)")) -> (appended path=w1166:path)
          n549 = case shown="20000, Default" w1161 {
            tunnel: w1166 -> [w1181 w1200 w1237 w1268]
            tunnel: w1169 -> [w1180 w1194 w1231 w1264]
            tunnel: [w1179 w1192 w1229 w1261] -> w1168
            tunnel: w1161 -> [_ w1188 w1225 _]
            tunnel: [w1173 w1184 w1221 w1259] -> w1159
            tunnel: [w1172 w1183 w1220 w1258] -> w1158
            tunnel: [FALSE TRUE TRUE TRUE] -> w1157
            frame 20000, Default {
              w1172 = -1.0
              n550 = local read "TX_PORT(t)"() -> (w1175:bool)
              n551 = Not(x=w1175) -> (.not. x?=w1174:bool)
              n552 = call-poly <vilib>:"Write Delimited Spreadsheet.vi"("file path (dialog if empty)"=w1181, "1D data"=w1180, "append to file? (new file:F)"=w1174) -> ("error out"=w1176:errorcluster)  [unwired: 11 in, 1 out]
              n553 = Format Into String(format string="%.3f", initial string="", error in=w1176, w1172) -> (resulting string=w1179:string, error out=w1173:errorcluster)
            }
            frame 25000 {
              n554 = Equal?(x=w1188, y=25000.0) -> (x = y?=w1185:bool)
              n555 = call-poly <vilib>:"Write Delimited Spreadsheet.vi"("file path (dialog if empty)"=w1200, "1D data"=w1194, "append to file? (new file:F)"=w1185) -> ("new file path (Not A Path if cancelled)"=w1198:path, "error out"=w1197:errorcluster)  [unwired: 11 in]
              n556 = Not(x=w1185) -> (.not. x?=w1186:bool)
              n557 = flat-sequence {
                tunnel: [w1203] -> w1199
                tunnel: w1198 -> [w1205]
                tunnel: w1197 -> [w1204]
                tunnel: [w1202] -> w1195
                tunnel: [w1201] -> w1189
                tunnel: w1199 -> [w1213]
                tunnel: [w1208] -> w1196
                tunnel: w1195 -> [w1208]
                tunnel: [w1207] -> w1183
                tunnel: [w1206] -> w1190
                tunnel: w1189 -> [w1206]
                tunnel: w1196 -> [w1218]
                tunnel: w1194 -> [w1217]
                tunnel: w1190 -> [w1216]
                tunnel: w1186 -> [w1215]
                tunnel: [w1214] -> w1184
                frame #0 {
                  n558 = call-poly <vilib>:"Read Delimited Spreadsheet.vi"("file path (dialog if empty)"=w1205, "error in (no error)"=w1204) -> ("new file path (Not A Path if cancelled)"=w1202:path, "all rows"=w1203:dbl[][], "error out"=w1201:errorcluster)  [unwired: 8 in, 3 out]
                }
                frame #1 {
                  n559 = Index Array(array=w1213, index (col)=1 ("disabled index (col)")) -> (element=w1212:dbl[])  [unwired: 1 in]
                  n560 = Array Max & Min(array=w1212) -> (max value=w1210:dbl, min value=w1209:dbl)  [unwired: 2 out]
                  n561 = Subtract(x=w1210, y=w1209) -> (x-y=w1207:dbl)
                  "lowband-flat" <- w1207
                }
                frame #2 {
                  # "open a new file"
                  n562 = call-poly <vilib>:"Write Delimited Spreadsheet.vi"("file path (dialog if empty)"=w1218, "1D data"=w1217, "append to file? (new file:F)"=w1215, "error in (no error)"=w1216) -> ("error out"=w1214:errorcluster)  [unwired: 10 in, 1 out]
                }
              }
              n563 = Format Into String(format string="%.3f", initial string="", w1183) -> (resulting string=w1192:string)  [unwired: 1 in, 1 out]
            }
            frame 32000 {
              n564 = Equal?(x=w1225, y=32000.0) -> (x = y?=w1222:bool)
              n565 = call-poly <vilib>:"Write Delimited Spreadsheet.vi"("file path (dialog if empty)"=w1237, "1D data"=w1231, "append to file? (new file:F)"=w1222) -> ("new file path (Not A Path if cancelled)"=w1235:path, "error out"=w1234:errorcluster)  [unwired: 11 in]
              n566 = Not(x=w1222) -> (.not. x?=w1223:bool)
              n567 = flat-sequence {
                tunnel: [w1240] -> w1236
                tunnel: w1235 -> [w1242]
                tunnel: w1234 -> [w1241]
                tunnel: [w1239] -> w1232
                tunnel: [w1238] -> w1226
                tunnel: w1236 -> [w1250]
                tunnel: [w1245] -> w1233
                tunnel: w1232 -> [w1245]
                tunnel: [w1244] -> w1220
                tunnel: [w1243] -> w1227
                tunnel: w1226 -> [w1243]
                tunnel: w1233 -> [w1255]
                tunnel: w1231 -> [w1254]
                tunnel: w1227 -> [w1253]
                tunnel: w1223 -> [w1252]
                tunnel: [w1251] -> w1221
                frame #0 {
                  n568 = call-poly <vilib>:"Read Delimited Spreadsheet.vi"("file path (dialog if empty)"=w1242, "error in (no error)"=w1241) -> ("new file path (Not A Path if cancelled)"=w1239:path, "all rows"=w1240:dbl[][], "error out"=w1238:errorcluster)  [unwired: 8 in, 3 out]
                }
                frame #1 {
                  n569 = Index Array(array=w1250, index (col)=1 ("disabled index (col)")) -> (element=w1249:dbl[])  [unwired: 1 in]
                  n570 = Array Max & Min(array=w1249) -> (max value=w1247:dbl, min value=w1246:dbl)  [unwired: 2 out]
                  n571 = Subtract(x=w1247, y=w1246) -> (x-y=w1244:dbl)
                  "lowband-flat 2" <- w1244
                }
                frame #2 {
                  # "open a new file"
                  n572 = call-poly <vilib>:"Write Delimited Spreadsheet.vi"("file path (dialog if empty)"=w1255, "1D data"=w1254, "append to file? (new file:F)"=w1252, "error in (no error)"=w1253) -> ("error out"=w1251:errorcluster)  [unwired: 10 in, 1 out]
                }
              }
              n573 = Format Into String(format string="%.3f", initial string="", w1220) -> (resulting string=w1229:string)  [unwired: 1 in, 1 out]
            }
            frame 40000 {
              n574 = call-poly <vilib>:"Write Delimited Spreadsheet.vi"("file path (dialog if empty)"=w1268, "1D data"=w1264, "append to file? (new file:F)"=TRUE) -> ("new file path (Not A Path if cancelled)"=w1266:path, "error out"=w1265:errorcluster)  [unwired: 11 in]
              n575 = flat-sequence {
                tunnel: [w1270] -> w1267
                tunnel: w1266 -> [w1272]
                tunnel: w1265 -> [w1271]
                tunnel: [w1269] -> w1260
                tunnel: w1267 -> [w1279]
                tunnel: [w1274] -> w1258
                tunnel: [w1273] -> w1259
                tunnel: w1260 -> [w1273]
                frame #0 {
                  n576 = call-poly <vilib>:"Read Delimited Spreadsheet.vi"("file path (dialog if empty)"=w1272, "error in (no error)"=w1271) -> ("all rows"=w1270:dbl[][], "error out"=w1269:errorcluster)  [unwired: 8 in, 4 out]
                }
                frame #1 {
                  n577 = Index Array(array=w1279, index (col)=1 ("disabled index (col)")) -> (element=w1278:dbl[])  [unwired: 1 in]
                  n578 = Array Max & Min(array=w1278) -> (max value=w1276:dbl, min value=w1275:dbl)  [unwired: 2 out]
                  n579 = Subtract(x=w1276, y=w1275) -> (x-y=w1274:dbl)
                  "hiband-flat" <- w1274
                }
              }
              n580 = Format Into String(format string="%.3f", initial string="", w1258) -> (resulting string=w1261:string)  [unwired: 1 in, 1 out]
            }
          }
        }
        frame #2 {
          n581 = Less Than 0?(x=w1285) -> (x < 0?=w1286:bool)
          n582 = case shown="False" w1286 {
            tunnel: [w1289 w1290] -> w1284
            tunnel: w1285 -> [w1289 w1291]
            frame False {
            }
            frame True {
              n583 = Negate(x=w1291) -> (-x=w1290:dbl)
            }
          }
          n584 = local read "tx_flat_lim"() -> (w1281:dbl)
          n585 = case shown="False" w1282 {
            tunnel: w1284 -> [_ w1294]
            tunnel: w1281 -> [_ w1295]
            tunnel: [TRUE w1296] -> w1283
            tunnel: [-1.0 w1294] -> w1280
            frame False {
            }
            frame True {
              n586 = Less?(x=w1294, y=w1295) -> (x < y?=w1296:bool)
            }
          }
          "Tx_Flat" <- w1280
        }
      }
      n587 = flat-sequence {
        tunnel: [w1344] -> w1151
        tunnel: [w1338] -> w1150
        tunnel: [w1334] -> w1149
        tunnel: [w1306] -> w1148
        tunnel: [w1324] -> w1147
        tunnel: [w1322] -> w1146
        tunnel: [w1315] -> w1142
        tunnel: [w1302] -> w1135
        tunnel: w1133 -> [w1300]
        tunnel: [w1299] -> w1130
        frame #0 {
          # "SPEC LIMITS"
          n588 = Boolean To (0,1)(Boolean=w1300) -> (0, 1=w1301:i16)
          n589 = local read "TX_PORT"() -> (w1298:i32)
          n590 = local read "ps_meas(i)(w)"() -> (w1351:dbl[])
          n591 = local read "MEAS_S11"() -> (w1333:bool)
          n592 = local read "s11_hsl"() -> (w1335:dbl)
          n593 = local read "h2_dbc"() -> (w1320:dbl)
          n594 = Equal To 0?(x=w1298) -> (x = 0?=w1297:bool)
          n595 = local read "MEAS_PS"() -> (w1332:bool)
          n596 = local read "pout_hsl"() -> (w1342:dbl)
          n597 = local read "pout_lsl"() -> (w1343:dbl)
          n598 = local read "fsl_ampl_corr"() -> (w1341:dbl)
          n599 = local read "dcw_hsl"() -> (w1348:dbl)
          n600 = local read "dcw_lsl"() -> (w1347:dbl)
          n601 = local read "h2_lim"() -> (w1319:dbl)
          n602 = local read "s11_lsl"() -> (w1310:dbl)
          n603 = local read "h2(t)"() -> (w1318:bool)
          n604 = local read "s11"() -> (w1311:dbl)
          n605 = Index Array(array=w1351, index=1) -> (element=w1349:dbl)
          n606 = case shown="True" w1332 {
            tunnel: w1349 -> [_ w1373]
            tunnel: w1348 -> [_ w1372]
            tunnel: w1347 -> [_ w1371]
            tunnel: [w1367 w1370] -> w1346
            tunnel: [w1367 w1369] -> w1345
            tunnel: [TRUE w1368] -> w1331
            frame False {
              w1367 = "-1"
            }
            frame True {
              n607 = Number To Fractional String(number=w1372) -> (F-format string=w1370:string)  [unwired: 3 in]
              n608 = In Range and Coerce(upper limit=w1372, x=w1373, lower limit=w1371) -> (In Range?=w1368:bool)  [unwired: 1 out]
              n609 = Number To Fractional String(number=w1371) -> (F-format string=w1369:string)  [unwired: 3 in]
            }
          }
          n610 = case shown="True" w1333 {
            tunnel: [w1375 w1381] -> w1337
            tunnel: [w1375 w1380] -> w1336
            tunnel: w1311 -> [_ w1378]
            tunnel: w1335 -> [_ w1377]
            tunnel: w1310 -> [_ w1379]
            tunnel: [TRUE w1376] -> w1329
            frame False {
              w1375 = "-1"
            }
            frame True {
              n611 = Number To Fractional String(number=w1377) -> (F-format string=w1380:string)  [unwired: 3 in]
              n612 = In Range and Coerce(upper limit=w1377, x=w1378, lower limit=w1379) -> (In Range?=w1376:bool)  [unwired: 1 out]
              n613 = Number To Fractional String(number=w1379) -> (F-format string=w1381:string)  [unwired: 3 in]
            }
          }
          n614 = case shown="True" w1318 {
            tunnel: w1320 -> [_ w1364]
            tunnel: w1319 -> [_ w1362]
            tunnel: [TRUE w1365] -> w1316
            tunnel: ["-1" w1363] -> w1315
            frame False {
            }
            frame True {
              n615 = Less?(x=w1364, y=w1362) -> (x < y?=w1365:bool)
              n616 = Number To Fractional String(number=w1362) -> (F-format string=w1363:string)  [unwired: 3 in]
            }
          }
          n617 = case shown="False" w1297 {
            tunnel: w1343 -> [w1357 _]
            tunnel: w1342 -> [w1356 _]
            tunnel: w1341 -> [w1355 _]
            tunnel: [w1354 w1359] -> w1340
            tunnel: [w1353 w1359] -> w1339
            tunnel: [w1352 TRUE] -> w1330
            frame False {
              n618 = Number To Fractional String(number=w1356) -> (F-format string=w1354:string)  [unwired: 3 in]
              n619 = In Range and Coerce(upper limit=w1356, x=w1355, lower limit=w1357) -> (In Range?=w1352:bool)  [unwired: 1 out]
              n620 = Number To Fractional String(number=w1357) -> (F-format string=w1353:string)  [unwired: 3 in]
            }
            frame True {
              w1359 = "-1"
            }
          }
          n621 = Build Array(w1346, w1345) -> (w1344:string[])
          n622 = Build Array(w1340, w1339) -> (w1338:string[])
          n623 = Build Array(w1336, w1337) -> (w1334:string[])
          n624 = Build Array(w1331, w1330, w1329, w1316, w1300) -> (w1328:bool[])
          n625 = Boolean To (0,1)(Boolean=w1331) -> (0, 1=w1325:i16)
          n626 = Boolean To (0,1)(Boolean=w1330) -> (0, 1=w1326:i16)
          n627 = Boolean To (0,1)(Boolean=w1329) -> (0, 1=w1327:i16)
          n628 = Boolean To (0,1)(Boolean=w1316) -> (0, 1=w1317:i16)
          n629 = And Array Elements(Boolean array=w1328) -> (logical AND=w1299:bool)
          n630 = Boolean To (0,1)(Boolean=w1299) -> (0, 1=w1323:i16)
          n631 = Format Into String(format string="%b%b%b%b%b", w1325, w1326, w1327, w1317, w1301) -> (resulting string=w1308:string, error out=w1313:errorcluster)  [unwired: 2 in]
          n632 = Format Into String(error in=w1313, w1323) -> (resulting string=w1324:string, error out=w1312:errorcluster)  [unwired: 2 in]
          n633 = Scan From String(format string="%5b", input string=w1308) -> (output 1=w1304:i32)  [unwired: 3 in, 3 out]
          n634 = local read "x > 0?"() -> (w1314:bool)
          n635 = Format Into String(format string="%d", w1304) -> (resulting string=w1302:string)  [unwired: 2 in, 1 out]
          n636 = Format Into String(format string="%d", error in=w1312, w1314) -> (resulting string=w1322:string)  [unwired: 1 in, 1 out]
          n637 = Format Into String(format string="%05b", w1304) -> (resulting string=w1306:string)  [unwired: 2 in, 1 out]
        }
      }
      n638 = global read "Test Parameter Globals_1.0.0.vi" "Global SN"() -> (w1143:string)
      n639 = local read "cmd;"() -> (w1144:string)
      n640 = local read "txp_#ofretries"() -> (w1129:i32)
      n641 = local read "readback"() -> (w1128:string)
      n642 = local read "result path"() -> (w1127:string)
      n643 = local read "temp 0x"() -> (w1145:string)
      "resulting string" <- w1135
    }
    frame #3 {
      n644 = Number To Decimal String(number=w1389) -> (decimal integer string=w1388:string)  [unwired: 1 in]
      n645 = case shown="True" TRUE {
        tunnel: [w1416 w1426] -> w1397
        tunnel: [w1413 w1425] -> w1396
        tunnel: w1395 -> [w1416 w1418]
        tunnel: ["-1" ("tx_p-f") w1417] -> w1394
        tunnel: w1393 -> [w1413 _]
        frame False {
          n646 = Select(t="PASS", s=w1413, f="FAIL") -> ()  [unwired: 1 out]
        }
        frame True {
          n647 = local read "ps_meas(i)(w)"() -> (w1420:dbl[])
          n648 = local read "fsl_ampl_corr"() -> (w1424:dbl)
          n649 = local read "Tx_Flat"() -> (w1423:dbl)
          n650 = local read "s11"() -> (w1422:dbl)
          n651 = Index Array(array=w1420, index=1) -> (element=w1421:dbl)
          n652 = call "Prod_Screen.vi"("pow_in"=w1421, "error in (no error)"=w1418, "s11_in"=w1422, "txflat_in"=w1423, "pout_in"=w1424) -> ("tx_p-f"=w1417:string, "TX-PASS?(T)"=w1425:bool, "error out"=w1426:errorcluster)  [unwired: 9 in, 3 out]
        }
      }
      "error out" <- w1397
      "TX-PASS?(T)" <- w1396
      n653 = Select(t=w1388, s=TRUE, f=w1391) -> (s? t:f=w1390:string)
      n654 = Insert Into Array(array=w1408, new element #1=w1407, new element #2=w1406, new element #3=w1390, new element #4=w1405, new element #5=w1404, new element #6=w1403, new element #7=w1402, new element #8=w1401, new element #9=w1400, new element #10=w1399, new element #11=w1398, new element #12=w1394, new element #13=w1386, new element #14=w1382) -> (w1384:string[])  [unwired: 1 in]
      n655 = Array Size(array=w1384) -> (size(s)=w1383:i32)
      n656 = for {
        N: w1383 -> [_]
        tunnel: w1384 -> [w1411] mode=indexing
        tunnel: [w1411] -> w1385 mode=indexing if=w1409
        n657 = Empty String/Path?(string/path=w1411) -> (empty?=w1410:bool)
        n658 = Not(x=w1410) -> (.not. x?=w1409:bool)
      }
      "Payload Results" <- w1385
      n659 = global write "Test Parameter Globals_1.0.0.vi" "Global_Pass(T)"(w1396) -> ()
    }
  }
